vi "TIM Control GUI_Modified for Testing.vi"() -> ()   [LabVIEW 2018]
doc: "This example demonstrates how to use the PID Design function to obtain PID parameters based on measured process."
uses:
  <vilib>/DAQmx/write.llb/DAQmx Write (Digital 1D Bool 1Chan 1Samp).vi
  <vilib>/DAQmx/read.llb/DAQmx Read (Analog 1D DBL NChan 1Samp).vi
  <vilib>/Instr/_visa.llb/VISA Configure Serial Port (Instr).vi
  <vilib>/DAQmx/create/channels.llb/DAQmx Create Channel (DO-Digital Output).vi
  <vilib>/DAQmx/miscellaneous.llb/DAQmx Fill In Error Info.vi
  <vilib>/addons/control/pid/pid.llb/PID Advanced (DBL).vi
  <vilib>/addons/control/pid/autopid.llb/PID Autotuning Design (Ziegler-Nichols).vi
  <vilib>/addons/control/pid/autopid.llb/PID Autotuning Design (Cohen-Coon).vi
  <vilib>/addons/control/pid/autopid.llb/PID Autotuning Design (Chien-Hrones-Reswick).vi
  <vilib>/addons/control/pid/autopid.llb/PID Autotuning Design (Internal Model Control).vi
  <vilib>/addons/control/pid/NI_PID_autopid.lvlib
  <vilib>/addons/control/pid/NI_PID_pid.lvlib
  <vilib>/ptbypt/NI_PtbyPt.lvlib
panel:
  out "Tracker 4 - X,Y,Z":cluster{"x":sgl, "y":sgl, "z":sgl}(graph)
  out "Tracker 3 - X,Y,Z":cluster{"x":sgl, "y":sgl, "z":sgl}(graph)
  out "Tracker 2 - X,Y,Z":cluster{"x":sgl, "y":sgl, "z":sgl}(graph)
  out "Tracker 1 - X,Y,Z":cluster{"x":sgl, "y":sgl, "z":sgl}(graph)
  in  "Set Point 1,5":dbl
  out "Real time Data 1,5,3,4":dbl[][](graph)
  in  "Set Point 2":dbl
  out "Real time Data 2":dbl[][](graph)
  in  "Set Point 7":dbl
  out "Real time Data 7":dbl[][](graph)
  in  "Set Point  6,8,9,10":dbl
  out "Real time Data 6,8,9,10":dbl[][](graph)
  in  "Set Point 11,12":dbl
  out "Real time Data -11,12":dbl[][](graph)
  out "error out":errorcluster {"code" format="%.0x"}
  in  "XYZAER":T1(array[cluster]) {"r" format="%1_6f"; "e" format="%1_6f"; "a" format="%1_6f"; "z" format="%1_6f"; "y" format="%1_6f"; "x" format="%1_6f"}
  out "Start Time Text":string
  out "Stop Time Text":string
  out "Elapsed Time Text":string
  out "HostFrameCount":u32
  out "Loop Iter":i32
  out "PnoData":bool
  in  "stop":bool
  out "?":bool
  in  "Muscle Control":T2(tab)=enum."M-11,12"
  out "Tuned PID gains 12":T3={"proportional gain (Kc)"=1.9838195929127882, "integral time (Ti, min)"=0.01995856284686879, "derivative time (Td, min)"=0.0} {"derivative time (Td, min)" format="%#.6g"; "integral time (Ti, min)" format="%#.6g"; "proportional gain (Kc)" format="%#.6g"}
  in  "Accept gain 12":bool
  in  "Control 12":T4(tab)
  in  "Ziegler-Nichols speed 12":u16(ring) items=["Fast", "Normal", "Slow"]
  in  "Tuning specifications 12":u16(ring) items=["Regulator - 0 %", "Regulator -  20%", "Servo - 0%", "Servo - 20%"]
  in  "Multiplicative factor 12":dbl(slide)=1.0 scale=0.01..100.0
  in  "Type of controller 12":u16(ring)=2 items=["P", "PI", "PID"]
  in  "Stop 12":bool
  in  "PID Gains 12":T3={"proportional gain (Kc)"=0.1625, "integral time (Ti, min)"=1.25, "derivative time (Td, min)"=0.0} {"derivative time (Td, min)" format="%#.6g"; "integral time (Ti, min)" format="%#.6g"; "proportional gain (Kc)" format="%#.6g"}
  in  "Autotune 12":bool
  in  "Reinitialize 12":bool
  in  "Excitation 12":dbl=0.5 format="%.2f"
  in  "Automatic 12":bool=TRUE
  in  "MV: 12":dbl(slide)=20.39115328927357 scale=-100.0..100.0
  out "PWM Output 12":bool
  in  "Median sample length 21":i32=100
  in  "INLET 1,5 ON/OFF 3":bool=TRUE
  out "Tuned PID gains 8":T3={"proportional gain (Kc)"=1.9838195929127882, "integral time (Ti, min)"=0.01995856284686879, "derivative time (Td, min)"=0.0} {"derivative time (Td, min)" format="%#.6g"; "integral time (Ti, min)" format="%#.6g"; "proportional gain (Kc)" format="%#.6g"}
  in  "Accept gain 8":bool
  in  "Control 8":T4(tab)
  in  "Ziegler-Nichols speed 8":u16(ring) items=["Fast", "Normal", "Slow"]
  in  "Tuning specifications 8":u16(ring) items=["Regulator - 0 %", "Regulator -  20%", "Servo - 0%", "Servo - 20%"]
  in  "Multiplicative factor 8":dbl(slide)=1.0 scale=0.01..100.0
  in  "Type of controller 8":u16(ring)=2 items=["P", "PI", "PID"]
  in  "Stop 8":bool
  in  "PID Gains 8":T3={"proportional gain (Kc)"=0.1625, "integral time (Ti, min)"=1.25, "derivative time (Td, min)"=0.0} {"derivative time (Td, min)" format="%#.6g"; "integral time (Ti, min)" format="%#.6g"; "proportional gain (Kc)" format="%#.6g"}
  in  "Autotune 8":bool
  in  "Reinitialize 8":bool
  in  "Excitation 8":dbl=0.5 format="%.2f"
  in  "Automatic 8":bool=TRUE
  in  "MV: 8":dbl(slide)=20.39115328927357 scale=-100.0..100.0
  out "PWM Output 8":bool
  in  "Median sample length 17":i32=100
  in  "INLET 2 ON/OFF 2":bool=TRUE
  out "Tuned PID gains 7":T3={"proportional gain (Kc)"=1.9838195929127882, "integral time (Ti, min)"=0.01995856284686879, "derivative time (Td, min)"=0.0} {"derivative time (Td, min)" format="%#.6g"; "integral time (Ti, min)" format="%#.6g"; "proportional gain (Kc)" format="%#.6g"}
  in  "Accept gain 7":bool
  in  "Control 7":T4(tab)
  in  "Ziegler-Nichols speed 7":u16(ring) items=["Fast", "Normal", "Slow"]
  in  "Tuning specifications 7":u16(ring) items=["Regulator - 0 %", "Regulator -  20%", "Servo - 0%", "Servo - 20%"]
  in  "Multiplicative factor 7":dbl(slide)=1.0 scale=0.01..100.0
  in  "Type of controller 7":u16(ring)=2 items=["P", "PI", "PID"]
  in  "Stop 7":bool
  in  "PID Gains 7":T3={"proportional gain (Kc)"=0.1625, "integral time (Ti, min)"=1.25, "derivative time (Td, min)"=0.0} {"derivative time (Td, min)" format="%#.6g"; "integral time (Ti, min)" format="%#.6g"; "proportional gain (Kc)" format="%#.6g"}
  in  "Autotune 7":bool
  in  "Reinitialize 7":bool
  in  "Excitation 7":dbl=0.5 format="%.2f"
  in  "Automatic 7":bool=TRUE
  in  "MV: 7":dbl(slide)=20.39115328927357 scale=-100.0..100.0
  out "PWM Output 7":bool
  in  "Median sample length 16":i32=100
  in  "INLET 7 ON/OFF 2":bool=TRUE
  out "Tuned PID gains 6":T3={"proportional gain (Kc)"=1.9838195929127882, "integral time (Ti, min)"=0.01995856284686879, "derivative time (Td, min)"=0.0} {"derivative time (Td, min)" format="%#.6g"; "integral time (Ti, min)" format="%#.6g"; "proportional gain (Kc)" format="%#.6g"}
  in  "Accept gain 6":bool
  in  "Control 6":T4(tab)
  in  "Ziegler-Nichols speed 6":u16(ring) items=["Fast", "Normal", "Slow"]
  in  "Tuning specifications 6":u16(ring) items=["Regulator - 0 %", "Regulator -  20%", "Servo - 0%", "Servo - 20%"]
  in  "Multiplicative factor 6":dbl(slide)=1.0 scale=0.01..100.0
  in  "Type of controller 6":u16(ring)=2 items=["P", "PI", "PID"]
  in  "Stop 6":bool
  in  "PID Gains 6":T3={"proportional gain (Kc)"=0.1625, "integral time (Ti, min)"=1.25, "derivative time (Td, min)"=0.0} {"derivative time (Td, min)" format="%#.6g"; "integral time (Ti, min)" format="%#.6g"; "proportional gain (Kc)" format="%#.6g"}
  in  "Autotune 6":bool
  in  "Reinitialize 6":bool
  in  "Excitation 6":dbl=0.5 format="%.2f"
  in  "Automatic 6":bool=TRUE
  in  "MV: 6":dbl(slide)=20.39115328927357 scale=-100.0..100.0
  out "PWM Output 6":bool
  in  "Median sample length 15":i32=100
  in  "INLET 6 ON/OFF 2":bool=TRUE
  in  "INLET":bool=TRUE
  out "PWM Output":bool
  in  "MV:":dbl(slide)=20.39115328927357 scale=-100.0..100.0
  in  "Median sample length":i32=100
  in  "Excitation":dbl=0.5 format="%.2f"
  in  "Type of controller":u16(ring)=2 items=["P", "PI", "PID"]
  in  "Control":T4(tab)
  in  "Ziegler-Nichols speed":u16(ring) items=["Fast", "Normal", "Slow"]
  in  "Tuning specifications":u16(ring) items=["Regulator - 0 %", "Regulator -  20%", "Servo - 0%", "Servo - 20%"]
  in  "Multiplicative factor":dbl(slide)=1.0 scale=0.01..100.0
  in  "Automatic":bool=TRUE
  in  "Reinitialize":bool
  in  "Accept gain":bool
  out "Tuned PID gains":T3={"proportional gain (Kc)"=1.9838195929127882, "integral time (Ti, min)"=0.01995856284686879, "derivative time (Td, min)"=0.0} {"derivative time (Td, min)" format="%#.6g"; "integral time (Ti, min)" format="%#.6g"; "proportional gain (Kc)" format="%#.6g"}
  in  "Autotune":bool
  in  "PID Gains":T3={"proportional gain (Kc)"=0.1625, "integral time (Ti, min)"=1.25, "derivative time (Td, min)"=0.0} {"derivative time (Td, min)" format="%#.6g"; "integral time (Ti, min)" format="%#.6g"; "proportional gain (Kc)" format="%#.6g"}
  in  "Stop":bool
  in  "M-11,12":i32=5
  in  "M-6,8,9,10":i32=5
  in  "M-7":i32=5
  in  "M-2":i32=5
  in  "M-1,5":i32=5
  out "Stimulus operating point 12":dbl=20.314221540357543
  out "Response operating point 12":dbl=51.08345461694337
  out "Identified Plant Parameters 12":T5={"Plant Gain (K)"=1.7609511324977591, "Time Constant (T)"=1.9621978490901302, "Dead Time (L)"=0.22467425343567116}
  out "Control Output 12":dbl[](graph)
  out "Measurement 12":dbl[](graph)
  out "Identified Plant Parameters":T5={"Plant Gain (K)"=1.7609511324977591, "Time Constant (T)"=1.9621978490901302, "Dead Time (L)"=0.22467425343567116}
  out "Control Output":dbl[](graph)
  out "Measurement":dbl[](graph)
  out "Stimulus operating point":dbl=20.314221540357543
  out "Response operating point":dbl=51.08345461694337
  out "Stimulus operating point 6":dbl=20.314221540357543
  out "Response operating point 6":dbl=51.08345461694337
  out "Identified Plant Parameters 6":T5={"Plant Gain (K)"=1.7609511324977591, "Time Constant (T)"=1.9621978490901302, "Dead Time (L)"=0.22467425343567116}
  out "Control Output 6":dbl[](graph)
  out "Measurement 6":dbl[](graph)
  out "Stimulus operating point 7":dbl=20.314221540357543
  out "Response operating point 7":dbl=51.08345461694337
  out "Identified Plant Parameters 7":T5={"Plant Gain (K)"=1.7609511324977591, "Time Constant (T)"=1.9621978490901302, "Dead Time (L)"=0.22467425343567116}
  out "Control Output 7":dbl[](graph)
  out "Measurement 7":dbl[](graph)
  out "Stimulus operating point 8":dbl=20.314221540357543
  out "Response operating point 8":dbl=51.08345461694337
  out "Identified Plant Parameters 8":T5={"Plant Gain (K)"=1.7609511324977591, "Time Constant (T)"=1.9621978490901302, "Dead Time (L)"=0.22467425343567116}
  out "Control Output 8":dbl[](graph)
  out "Measurement 8":dbl[](graph)
  out "Connected":bool
  out "Running":bool
  out "Position Sensor Data":cluster{dbl, "x":sgl}[](graph)
  out "Sensor Raw Value 2":i32
  in  "COM Port-Sensor 2":refnum<visa-resource-name>="COM5"
  in  "upper/lower infle":enum32{"Page 1", "Page 2"}(tab)
  out "Force in Kilograms":dbl(graph)
  out "Force in Newtons":dbl(graph)
  in  "lower/upper infle":enum32{"Page 1", "Page 2"}(tab)
  out "Force in Newtons 2":dbl(graph)
  out "Force in Kilograms 2":dbl(graph)
  in  "COM Port-Sensor 1":refnum<visa-resource-name>="COM4"
  out "Sensor Raw Value":i32
  in  "Tab Control":T6(tab)
  in  "Instructions":string="Overview: This example demonstrates how to use the PID Autotuning Design to obtain PID parameters based on setpoint and process variable collected in another loop.\nInstructions:\n1. Run the VI and wait until the process variable (PV) reaches near setpoint (SP).\n2.  In the PID Autotuning Design section, select the type of algorithm, type of controller and excitation amplitude for the 'open loop step response'. Then, click Autotune to start the process. Select the Identified Plant Parameter tab and see the results from the identification.\n3.  When the tuned PID gains do not change anymore, the identification is done and you have the option to accept by clicking Accept gain, which will transfer the new gain to PID Gains.\n4. Click the Autotune button again to go back to the automatic control state. You can try different options and repeat this process.\n5. Click Stop to stop the VI.\n"
  # "Pressure Alarm"
  # "Force Sensor Data"
  # "Position Sensor Data"
  # "PID Controller"
  # "PID Autotuning Design"
  # "No additional parameters"
  # "PID Controller"
  # "PID Autotuning Design"
  # "PID Controller"
  # "PID Autotuning Design"
  # "No additional parameters"
  # "PID Controller"
  # "PID Autotuning Design"
  # "No additional parameters"
  # "PID Controller"
  # "PID Autotuning Design"
  # "No additional parameters"
  # "Muscle Control"
  # "PID Controller"
  # "PID Autotuning Design"
  # "No additional parameters"
  # "Pressure Cut Off to trigger the alarm"
  # "M-11,12"
  # "M-3,4"
  # "M-1,5"
  # "M-6,8,9,10"
  # "M-7"
  # "M-2"
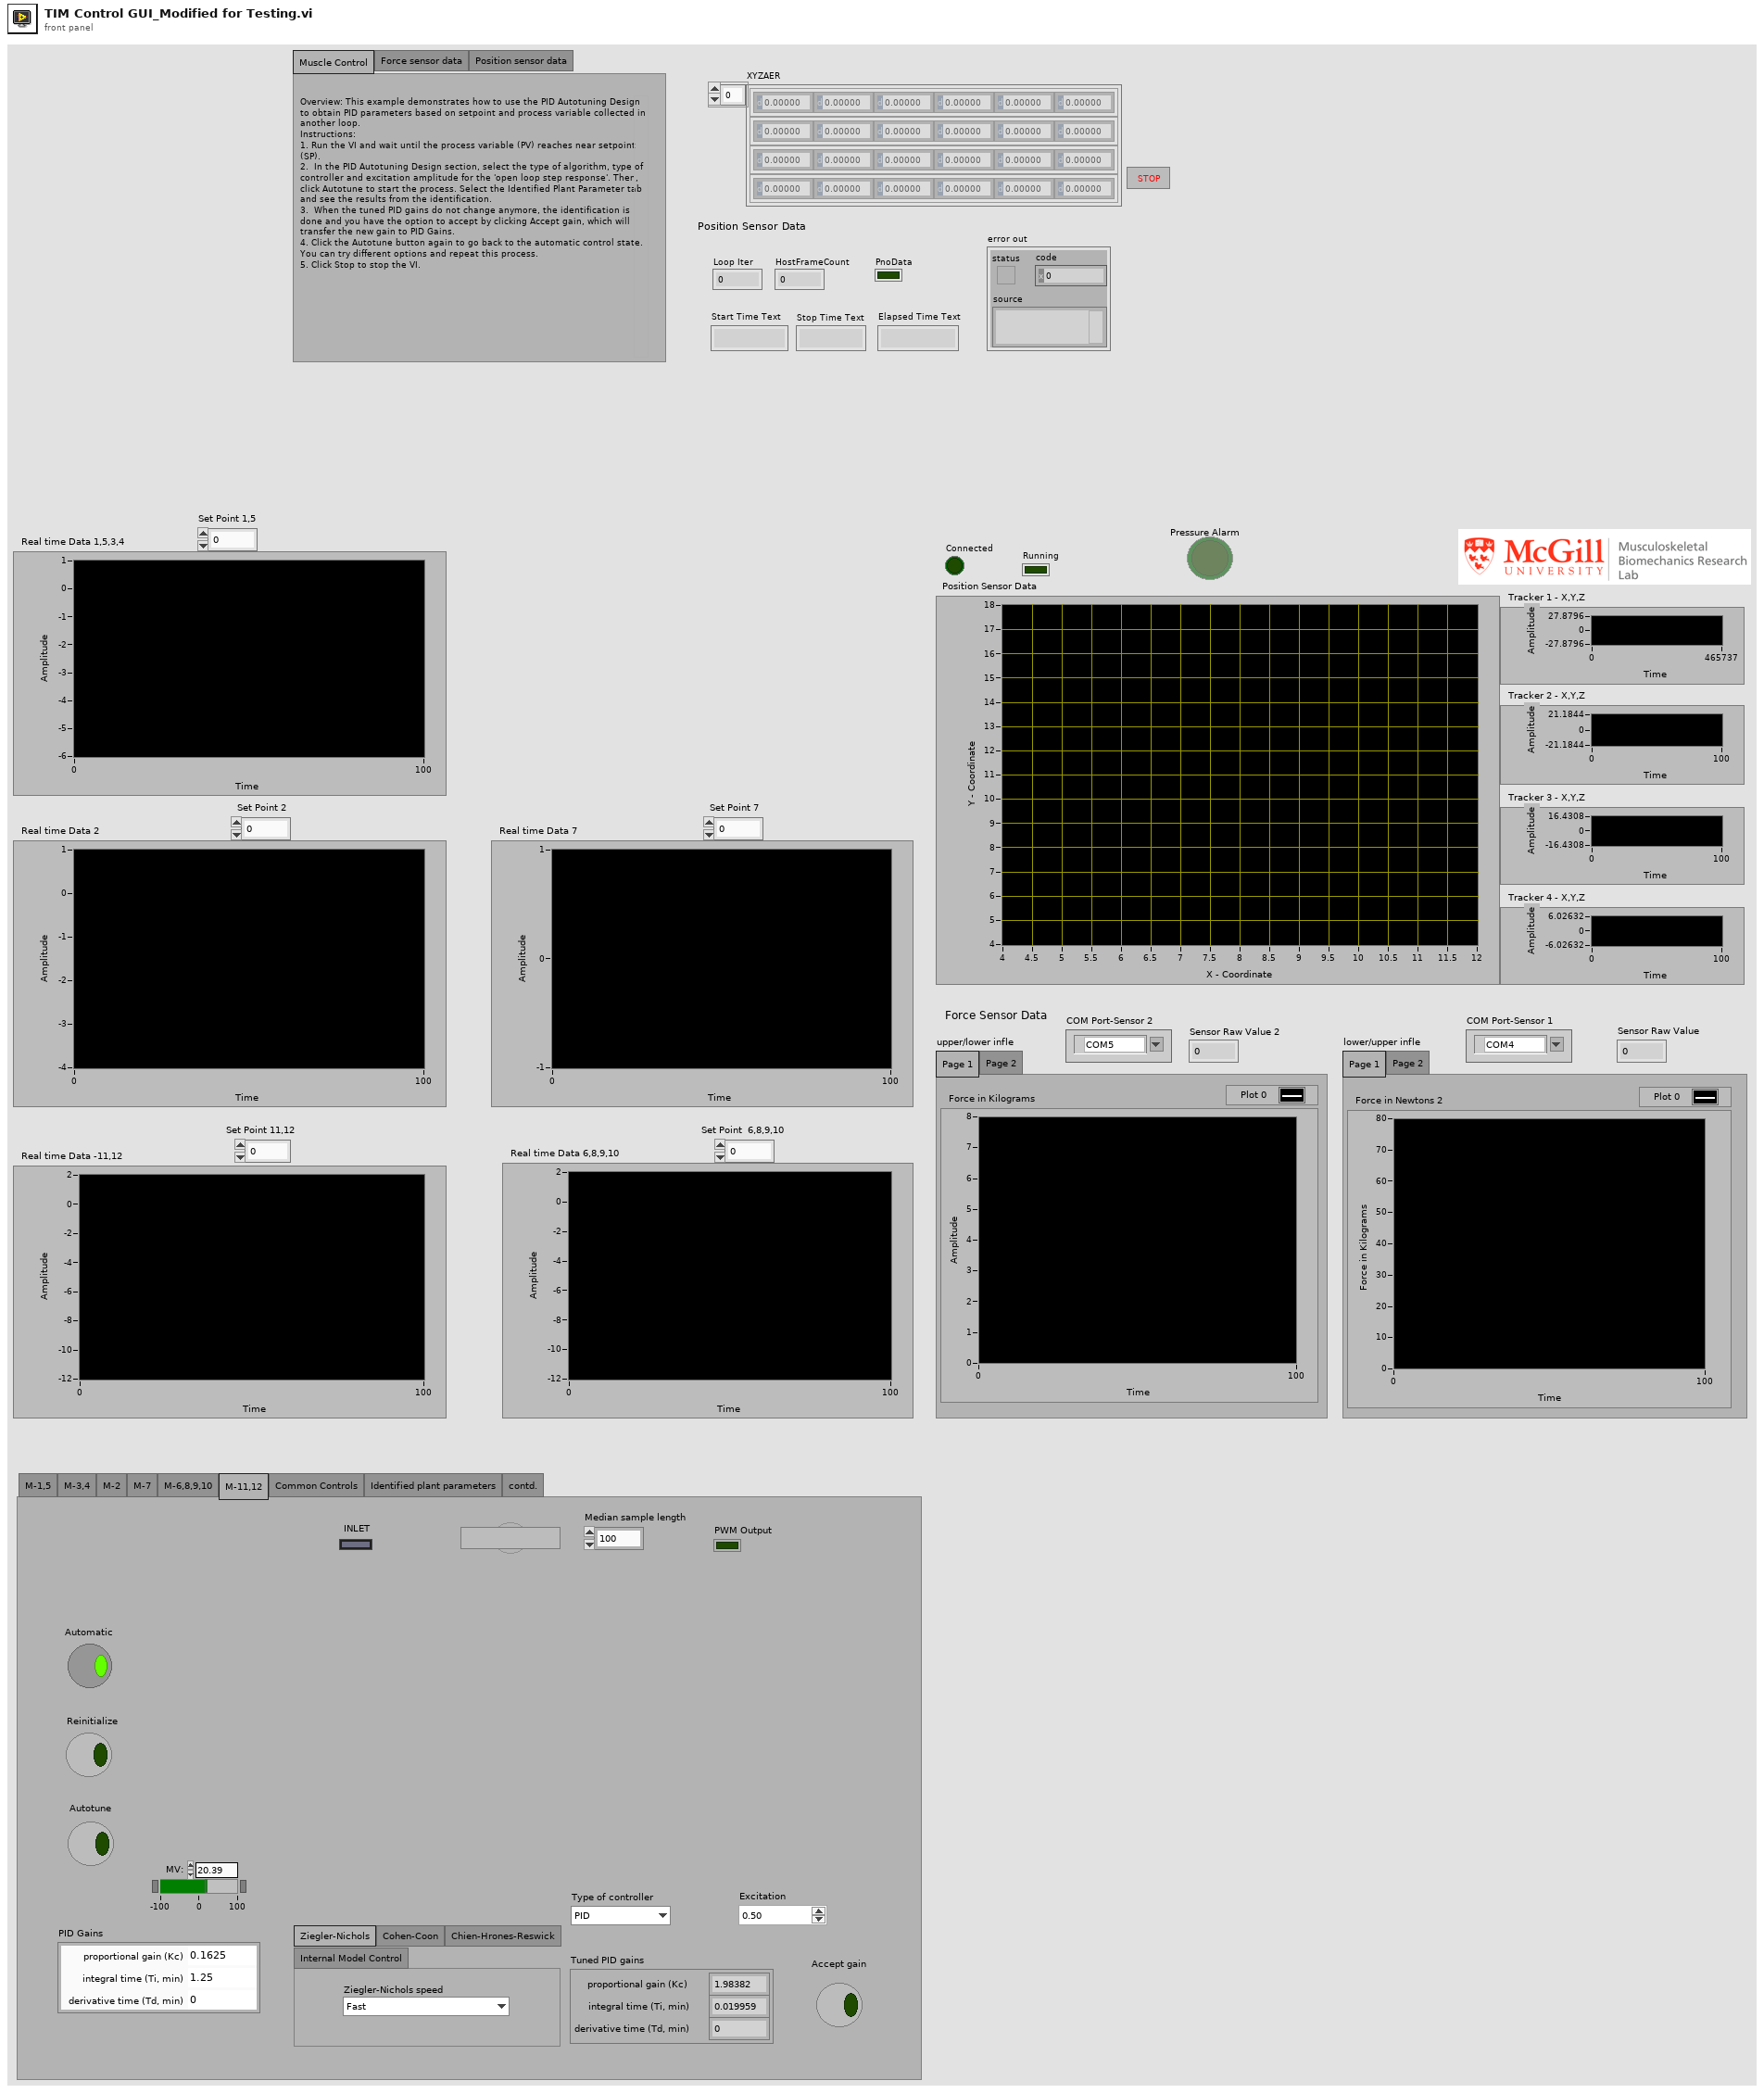
[diagram p1: front panel]
types:
  T1 = cluster{"x":sgl, "y":sgl, "z":sgl, "a":sgl, "e":sgl, "r":sgl}[]
  T2 = enum32{"M-1,5", "M-3,4", "M-2", "M-7", "M-6,8,9,10", "M-11,12", "Common Controls", "Identified plant parameters", "contd."}
  T3 = cluster{"proportional gain (Kc)":dbl, "integral time (Ti, min)":dbl, "derivative time (Td, min)":dbl}
  T4 = enum32{"Ziegler-Nichols", "Cohen-Coon", "Chien-Hrones-Reswick", "Internal Model Control"}
  T5 = cluster{"Plant Gain (K)":dbl, "Time Constant (T)":dbl, "Dead Time (L)":dbl}
  T6 = enum32{"Muscle Control", "Force sensor data", "Position sensor data"}
  T7 = cluster{"static gain":dbl, "lag (s)":dbl, "deadtime (s)":dbl, "load":dbl, "deadband":dbl, "sensor noise":dbl, "initial PV":dbl, "plant noise":dbl}
  T8 = cluster{"x":sgl, "y":sgl, "z":sgl, "a":sgl, "e":sgl, "r":sgl}
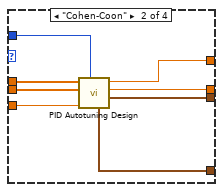
[diagram p2: hidden frame]
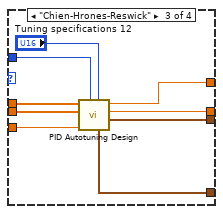
[diagram p3: hidden frame]
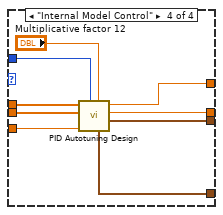
[diagram p4: hidden frame]
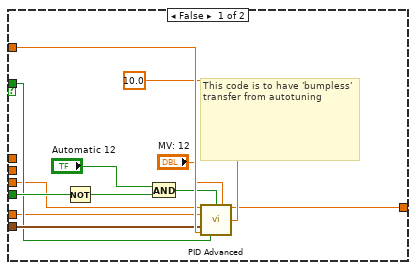
[diagram p6: hidden frame]
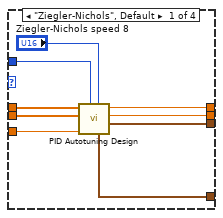
[diagram p7: hidden frame]
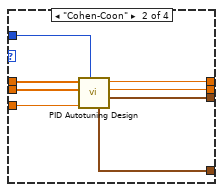
[diagram p8: hidden frame]
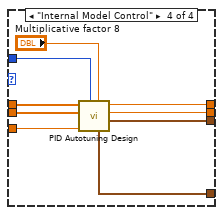
[diagram p9: hidden frame]
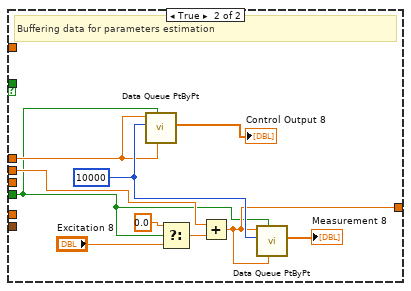
[diagram p11: hidden frame]
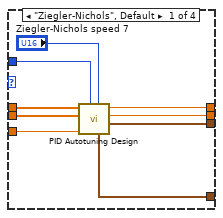
[diagram p12: hidden frame]
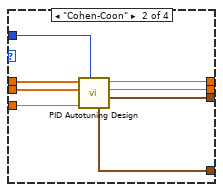
[diagram p13: hidden frame]
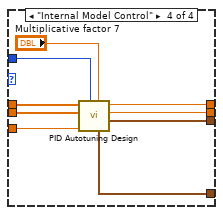
[diagram p14: hidden frame]
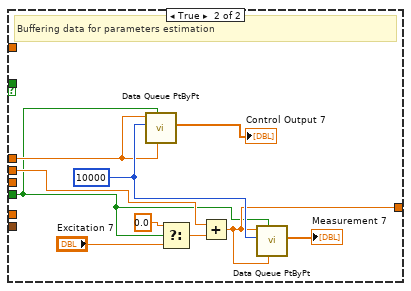
[diagram p16: hidden frame]
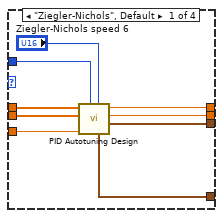
[diagram p17: hidden frame]
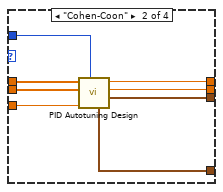
[diagram p18: hidden frame]
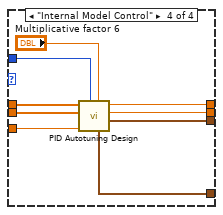
[diagram p19: hidden frame]
diagram:
  w16 = 0.0 ("output")
  w19 = FALSE ("Stop")
  w22 = 0.0 ("output")
  w25 = FALSE ("Stop")
  w28 = 0.0 ("output")
  w31 = FALSE ("Stop")
  w34 = 0.0 ("output")
  w37 = FALSE ("Stop")
  w42 = 2400  # BufferFrameCount
  w76 = 0.0 ("output")
  w79 = FALSE ("Stop")
  # "Muscle-1,5 PID CONTROL LOOP (Auto Tuning)"
  # "Muscle-2 PID CONTROL LOOP (Auto Tuning)"
  # "Muscle-7 PID CONTROL LOOP (Auto Tuning)"
  # "Muscle-6,8,9,10 PID CONTROL LOOP (Auto Tuning)"
  # "Muscle-11,12 PID CONTROL LOOP (Auto Tuning)"
  # "FORCE SENSOR CONTROL LOOP"
  # "POSITION SENSOR CONTROL LOOP"
  # "Pressure Alarm"
  # "8. Close Tracker connection."
  # "3. Query Max num sensors supported by the tracker."
  # "4. Allocate raw buffer to hold 2400 frames of data."
  # "5. Start Continuous mode."
  # "7. Stop Continuous mode."
  # "6. Start the loop. Loop exits when Stop Button is hit."
  n1 = Obtain Queue(element data type=0.0) -> (queue out=w11:refnum<queue>)  [unwired: 4 in, 2 out]
  n2 = while {
    shift-left: 0.0 ("Plant Output") -> [w195]
    shift-right: [w190] -> _
    tunnel: w37 -> [_]
    shift-right: [w176] -> _
    shift-left: 0.01 -> [w174]
    shift-right: [w149] -> _
    shift-left: TRUE -> [w173]
    shift-right: [w151] -> _
    shift-left: w34 -> [w172]
    shift-right: [w175] -> _
    shift-left: w34 -> [w171]
    tunnel: [w146] -> w33
    tunnel: [w133] -> w3
    tunnel: w11 -> [w131]
    stop <- "Stop 6" stop-if-true
    w84 = 1 items=["one channel for each line", "one channel for all lines"] ("line grouping")
    w92 = 1 items=["one channel for each line", "one channel for all lines"] ("line grouping")
    w100 = 1 items=["one channel for each line", "one channel for all lines"] ("line grouping")
    w108 = 1 items=["one channel for each line", "one channel for all lines"] ("line grouping")
    w116 = 1 items=["one channel for each line", "one channel for all lines"] ("line grouping")
    w124 = 1 items=["one channel for each line", "one channel for all lines"] ("line grouping")
    w137 = 1 items=["one channel for each line", "one channel for all lines"] ("line grouping")
    w146 = 0.05 ("Sampling Time dt (s)")
    w154 = 1 items=["one channel for each line", "one channel for all lines"] ("line grouping")
    w162 = 0.5 ("x")
    w189 = T7 {"static gain"=2.5, "lag (s)"=2.5, "deadtime (s)"=0.01, "load"=0.0, "deadband"=0.0, "sensor noise"=0.0, "initial PV"=30.0, "plant noise"=0.0}  # Process parameters
    w191 = FALSE  # Integrator ?
    # "Inlet 11"
    # "Exhaust 10"
    # "Inlet 11"
    # "Exhaust 9"
    # "Inlet 11"
    # "Exhaust 8"
    # "C."
    # "Inlet 11"
    # "Exhaust 6"
    # "B."
    # "A."
    # "A.Output to PWM Logic \nB. Simulated Plant\nC. Draw Chart"
    # "Main PID Loop Control"
    n3 = Dequeue Element(queue=w131) -> (element=w132:dbl)  [unwired: 2 in, 3 out]
    n4 = Multiply(x=w146, y=1000.0) -> (x*y=w188:dbl)
    n5 = Not(x="Autotune 6") -> (.not. x?=w192:bool)
    n6 = feedback #1() -> (w197:bool)  [unwired: 1 in]
    n7 = feedback-in #1("Autotune 6") -> ()
    n8 = Wait Until Next ms Multiple(millisecond multiple=w188) -> ()  [unwired: 1 out]
    n9 = Exclusive Or(1:w197, 2:"Autotune 6") -> (0:w196:bool)
    n10 = feedback #2() -> (w194:dbl)  [unwired: 1 in]
    n11 = Multiply(x=w132, y=-1000.0) -> (x*y=w178:dbl)
    n12 = call <vilib>:"Median PtByPt.vi"("sample length"="Median sample length 15", "x"=w178) -> ("median"=w177:dbl)  [unwired: 2 in, 1 out]
    n13 = Square(x=w177) -> (x^2=w185:dbl)
    n14 = Multiply(x=w177, y=16.572) -> (x*y=w181:dbl)
    n15 = Multiply(x=w185, y=-0.06) -> (x*y=w182:dbl)
    n16 = Add(x=w181, y=w182) -> (x+y=w180:dbl)
    n17 = Add(x=-1011.3, y=w180) -> (x+y=w144:dbl)
    n18 = case shown="False" "Autotune 6" {
      tunnel: w146 -> [w212 _]
      tunnel: [w201 w217] -> w151
      tunnel: w195 -> [_ w216]
      tunnel: "PID Gains 6" -> [w211 _]
      tunnel: "Reinitialize 6" -> [w208 _]
      tunnel: w196 -> [w210 w215]
      tunnel: w194 -> [_ w219]
      tunnel: w144 -> [w204 _]
      tunnel: "Set Point  6,8,9,10" -> [w203 _]
      frame False {
        # "This code is to have 'bumpless' transfer from autotuning"
        n19 = Not(x=w210) -> (.not. x?=w207:bool)
        n20 = And(x="Automatic 6", y=w207) -> (x .and. y?=w209:bool)
        n21 = call-poly <vilib>:"PID Advanced.vi"("setpoint"=w203, "auto? (T)"=w209, "manual control"="MV: 6", "process variable"=w204, "alpha"=10.0, "PID gains"=w211, "dt (s)"=w212, "reinitialize? (F)"=w208) -> ("output"=w201:dbl)  [unwired: 6 in, 1 out]
      }
      frame True {
        w222 = 10000 ("sample length")
        # "Buffering data for parameters estimation"
        n22 = call <vilib>:"Data Queue PtByPt.vi"("initial queue element"=w216, "initialize"=w215, "sample length"=w222, "input data point"=w216) -> ("Current Queue"=→"Control Output 6":dbl[])  [unwired: 3 in, 4 out]
        n23 = Select(t=0.0, s=w215, f="Excitation 6") -> (s? t:f=w220:dbl)
        n24 = Add(x=w219, y=w220) -> (x+y=w217:dbl)
        n25 = call <vilib>:"Data Queue PtByPt.vi"("initial queue element"=w217, "initialize"=w215, "sample length"=w222, "input data point"=w217) -> ("Current Queue"=→"Measurement 6":dbl[])  [unwired: 3 in, 4 out]
      }
    }
    n26 = feedback-in #2(w151, w192) -> ()
    n27 = Greater?(x=w144, y="M-6,8,9,10") -> (0:w133:bool)
    n28 = Add(x=w174, y=w162) -> (x+y=w163:dbl)
    n29 = Subtract(x=w174, y=w162) -> (x-y=w161:dbl)
    n30 = Equal?(x=w172, y=w151) -> (x = y?=w169:bool)
    n31 = Greater?(x=w151, y=w172) -> (0:w168:bool)
    n32 = Select(t=w173, s=w169, f=w168) -> (s? t:f=w149:bool)
    "PWM Output 6" <- w149
    n33 = call "Plant System.vi"("Integrator ?"=w191, "Plant Input"=w151, "dt (s)"=w146, "process parameters"=w189) -> ("Plant Output"=w190:dbl)  [unwired: 11 in]
    n34 = Increment(x="Set Point  6,8,9,10") -> (x+1=w167:dbl)
    n35 = Decrement(x="Set Point  6,8,9,10") -> (x-1=w166:dbl)
    n36 = Select(t=w163, s=w149, f=w161) -> (s? t:f=w176:dbl)
    n37 = call-poly <vilib>:"DAQmx Create Virtual Channel.vi"("lines"=tag "cDAQ1Mod1/port0/line3", "line grouping"=w108) -> ("task out"=w110:refnum<k21>, "error out"=w109:errorcluster)  [unwired: 12 in]
    n38 = call-poly <vilib>:"DAQmx Create Virtual Channel.vi"("lines"=tag "cDAQ1Mod2/port0/line3", "line grouping"=w100) -> ("task out"=w102:refnum<k21>, "error out"=w101:errorcluster)  [unwired: 12 in]
    n39 = Select(t=w167, s=w149, f=w166) -> (s? t:f=w165:dbl)
    n40 = Not(x=w149) -> (.not. x?=w148:bool)
    n41 = call-poly <vilib>:"DAQmx Create Virtual Channel.vi"("lines"=tag "cDAQ1Mod1/port0/line4", "line grouping"=w154) -> ("task out"=w156:refnum<k21>, "error out"=w155:errorcluster)  [unwired: 12 in]
    n42 = call-poly <vilib>:"DAQmx Create Virtual Channel.vi"("lines"=tag "cDAQ1Mod2/port0/line4", "line grouping"=w137) -> ("task out"=w139:refnum<k21>, "error out"=w138:errorcluster)  [unwired: 12 in]
    n43 = Build Array(w144, "Set Point  6,8,9,10", w165) -> (w164:dbl[])
    n44 = Initialize Array("INLET 6 ON/OFF 2", 1 ("dimension size")) -> (w81:bool[])
    n45 = Initialize Array(w148, 1 ("dimension size")) -> (w82:bool[])
    n46 = local write "MV: 6"(w151) -> ()
    n47 = Add(x=w171, y=w174) -> (x+y=w175:dbl)
    n48 = Build Array(w164) -> (→"Real time Data 6,8,9,10":dbl[][])
    n49 = call-poly <vilib>:"DAQmx Write.vi"("task/channels in"=w110, "auto start"=TRUE, "data"=w82, "error in"=w109) -> ("task out"=w112:refnum<k21>, "error out"=w113:errorcluster)  [unwired: 9 in, 1 out]
    n50 = call-poly <vilib>:"DAQmx Write.vi"("task/channels in"=w102, "auto start"=TRUE, "data"=w81, "error in"=w101) -> ("task out"=w104:refnum<k21>, "error out"=w105:errorcluster)  [unwired: 9 in, 1 out]
    n51 = call-poly <vilib>:"DAQmx Write.vi"("task/channels in"=w156, "auto start"=TRUE, "data"=w82, "error in"=w155) -> ("task out"=w158:refnum<k21>, "error out"=w159:errorcluster)  [unwired: 9 in, 1 out]
    n52 = call-poly <vilib>:"DAQmx Write.vi"("task/channels in"=w139, "auto start"=TRUE, "data"=w81, "error in"=w138) -> ("task out"=w141:refnum<k21>, "error out"=w142:errorcluster)  [unwired: 9 in, 1 out]
    n53 = call <vilib>:"DAQmx Clear Task.vi"("task in"=w112, "error in"=w113) -> ("error out"=w107:errorcluster)  [unwired: 13 in]
    n54 = call <vilib>:"DAQmx Clear Task.vi"("task in"=w104, "error in"=w105) -> ("error out"=w99:errorcluster)  [unwired: 13 in]
    n55 = call <vilib>:"DAQmx Clear Task.vi"("task in"=w158, "error in"=w159) -> ("error out"=w153:errorcluster)  [unwired: 13 in]
    n56 = call <vilib>:"DAQmx Clear Task.vi"("task in"=w141, "error in"=w142) -> ("error out"=w136:errorcluster)  [unwired: 13 in]
    n57 = call <vilib>:"Simple Error Handler.vi"("error in (no error)"=w107) -> ()  [unwired: 4 in, 5 out]
    n58 = call <vilib>:"Simple Error Handler.vi"("error in (no error)"=w99) -> ()  [unwired: 4 in, 5 out]
    n59 = call <vilib>:"Simple Error Handler.vi"("error in (no error)"=w153) -> ()  [unwired: 4 in, 5 out]
    n60 = call <vilib>:"Simple Error Handler.vi"("error in (no error)"=w136) -> ()  [unwired: 4 in, 5 out]
    n61 = call-poly <vilib>:"DAQmx Create Virtual Channel.vi"("lines"=tag "cDAQ1Mod8/port0/line6", "line grouping"=w92) -> ("task out"=w94:refnum<k21>, "error out"=w93:errorcluster)  [unwired: 12 in]
    n62 = call-poly <vilib>:"DAQmx Create Virtual Channel.vi"("lines"=tag "cDAQ1Mod7/port0/line5", "line grouping"=w84) -> ("task out"=w86:refnum<k21>, "error out"=w85:errorcluster)  [unwired: 12 in]
    n63 = call-poly <vilib>:"DAQmx Create Virtual Channel.vi"("lines"=tag "cDAQ1Mod8/port0/line3", "line grouping"=w124) -> ("task out"=w126:refnum<k21>, "error out"=w125:errorcluster)  [unwired: 12 in]
    n64 = call-poly <vilib>:"DAQmx Create Virtual Channel.vi"("lines"=tag "cDAQ1Mod7/port0/line2", "line grouping"=w116) -> ("task out"=w118:refnum<k21>, "error out"=w117:errorcluster)  [unwired: 12 in]
    n65 = call-poly <vilib>:"DAQmx Write.vi"("task/channels in"=w94, "auto start"=TRUE, "data"=w82, "error in"=w93) -> ("task out"=w96:refnum<k21>, "error out"=w97:errorcluster)  [unwired: 9 in, 1 out]
    n66 = call-poly <vilib>:"DAQmx Write.vi"("task/channels in"=w86, "auto start"=TRUE, "data"=w81, "error in"=w85) -> ("task out"=w88:refnum<k21>, "error out"=w89:errorcluster)  [unwired: 9 in, 1 out]
    n67 = call-poly <vilib>:"DAQmx Write.vi"("task/channels in"=w126, "auto start"=TRUE, "data"=w82, "error in"=w125) -> ("task out"=w128:refnum<k21>, "error out"=w129:errorcluster)  [unwired: 9 in, 1 out]
    n68 = call-poly <vilib>:"DAQmx Write.vi"("task/channels in"=w118, "auto start"=TRUE, "data"=w81, "error in"=w117) -> ("task out"=w120:refnum<k21>, "error out"=w121:errorcluster)  [unwired: 9 in, 1 out]
    n69 = call <vilib>:"DAQmx Clear Task.vi"("task in"=w96, "error in"=w97) -> ("error out"=w91:errorcluster)  [unwired: 13 in]
    n70 = call <vilib>:"DAQmx Clear Task.vi"("task in"=w88, "error in"=w89) -> ("error out"=w83:errorcluster)  [unwired: 13 in]
    n71 = call <vilib>:"DAQmx Clear Task.vi"("task in"=w128, "error in"=w129) -> ("error out"=w123:errorcluster)  [unwired: 13 in]
    n72 = call <vilib>:"DAQmx Clear Task.vi"("task in"=w120, "error in"=w121) -> ("error out"=w115:errorcluster)  [unwired: 13 in]
    n73 = call <vilib>:"Simple Error Handler.vi"("error in (no error)"=w91) -> ()  [unwired: 4 in, 5 out]
    n74 = call <vilib>:"Simple Error Handler.vi"("error in (no error)"=w83) -> ()  [unwired: 4 in, 5 out]
    n75 = call <vilib>:"Simple Error Handler.vi"("error in (no error)"=w123) -> ()  [unwired: 4 in, 5 out]
    n76 = call <vilib>:"Simple Error Handler.vi"("error in (no error)"=w115) -> ()  [unwired: 4 in, 5 out]
  }
  n77 = local write "Stop 6"(w37) -> ()
  n78 = while {
    tunnel: w37 -> [_]
    tunnel: w33 -> [w226]
    stop <- w236 stop-if-true
    # "If dT and deadtime have similar values, the identification could evaluate deadtime as zero and this generates proportional gain equal to Inf. This code avoid gain changes in this situations."
    # "Autotuning Loop"
    n79 = local read "Control Output 6"() -> (w238:dbl[])
    n80 = local read "Measurement 6"() -> (w237:dbl[])
    n81 = case shown="\"Chien-Hrones-Reswick\"" "Control 6" {
      tunnel: w238 -> [w247 w255 w264 w273]
      tunnel: w237 -> [w246 w254 w263 w272]
      tunnel: [w245 w253 w262 w271] -> w225
      tunnel: [w244 w252 w261 w270] -> w224
      tunnel: w226 -> [w243 w251 w260 w269]
      tunnel: [w242 w250 w259 w268] -> w223
      tunnel: [w241 w249 w258 w267] -> w228
      tunnel: "Type of controller 6" -> [w240 w248 w257 w266]
      frame "Ziegler-Nichols", Default {
        n82 = call-poly <vilib>:"PID Autotuning Design.vi"("Ziegler-Nichols Speed"="Ziegler-Nichols speed 6", "Type of Controller"=w240, "dt (s)"=w243, "Response signal"=w246, "Stimulus signal"=w247) -> ("PID gains"=w241:T3, "response operating point"=w244:dbl, "stimulus operating point"=w245:dbl, "Plant Parameters"=w242:T5)  [unwired: 3 in]
      }
      frame "Cohen-Coon" {
        n83 = call-poly <vilib>:"PID Autotuning Design.vi"("Type of Controller"=w248, "dt (s)"=w251, "Response signal"=w254, "Stimulus signal"=w255) -> ("PID gains"=w249:T3, "response offset"=w252:dbl, "stimulus offset"=w253:dbl, "Plant Parameters"=w250:T5)  [unwired: 4 in]
      }
      frame "Chien-Hrones-Reswick" {
        n84 = call-poly <vilib>:"PID Autotuning Design.vi"("Tuning specifications"="Tuning specifications 6", "Type of Controller"=w257, "dt (s)"=w260, "Response signal"=w263, "Stimulus signal"=w264) -> ("PID gains"=w258:T3, "response offset"=w261:dbl, "stimulus offset"=w262:dbl, "Plant Parameters"=w259:T5)  [unwired: 3 in]
      }
      frame "Internal Model Control" {
        n85 = call-poly <vilib>:"PID Autotuning Design.vi"("Desired Time Constant (tau_c)"="Multiplicative factor 6", "Type of Controller"=w266, "dt (s)"=w269, "Response signal"=w272, "Stimulus signal"=w273) -> ("PID gains"=w267:T3, "response offset"=w270:dbl, "stimulus offset"=w271:dbl, "Plant Parameters"=w268:T5)  [unwired: 3 in]
      }
    }
    "Stimulus operating point 6" <- w225
    "Response operating point 6" <- w224
    "Identified Plant Parameters 6" <- w223
    n86 = Unbundle(w228) -> ("proportional gain (Kc)"=w231:dbl)  [unwired: 2 out]
    n87 = Equal?(x=w231, y=inf) -> (x = y?=w230:bool)
    n88 = feedback #3() -> (w229:T3)  [unwired: 1 in]
    n89 = Select(t=w229, s=w230, f=w228) -> (s? t:f=w227:T3)
    "Tuned PID gains 6" <- w227
    n90 = feedback-in #3(w227) -> ()
    n91 = case shown="True" "Accept gain 6" {
      tunnel: w227 -> [_ w274]
      frame False {
      }
      frame True {
        n92 = local write "PID Gains 6"(w274) -> ()
      }
    }
    n93 = local read "Stop 6"() -> (w236:bool)
  }
  n94 = local write "Stop"(w79) -> ()
  n95 = call-poly "VISA Configure Serial Port"("VISA resource name"="COM Port-Sensor 1") -> ("VISA resource name out"=w70:refnum<visa-resource-name>, "error out"=w69:errorcluster)  [unwired: 9 in, 4 out]
  n96 = call-poly "VISA Configure Serial Port"("VISA resource name"="COM Port-Sensor 2") -> ("VISA resource name out"=w65:refnum<visa-resource-name>, "error out"=w64:errorcluster)  [unwired: 9 in, 4 out]
  n97 = while {
    shift-right: [w282] -> w71
    shift-left: w70 -> [w278]
    tunnel: w69 -> [w277]
    tunnel: [w279] -> w72
    stop <- w280 stop-if-true
    # "Serial Read Loop"
    n98 = case shown="True" TRUE {
      tunnel: [w294 w298] -> w282
      tunnel: w278 -> [w296 w298]
      tunnel: [w293 w297] -> w279
      tunnel: w277 -> [w295 w297]
      frame True {
        n99 = VISA Read(VISA resource name=w296, byte count=u32 1000, error in (no error)=w295) -> (VISA resource name out=w294:refnum<visa-resource-name>, read buffer=w291:string, error out=w293:errorcluster)  [unwired: 1 out]
        n100 = Decimal String To Number(string=w291) -> (number=w289:i32)  [unwired: 2 in, 1 out]
        "Sensor Raw Value" <- w289
        n101 = call <vilib>:"Median PtByPt.vi"("sample length"=20, "x"=w289) -> ("median"=w287:dbl)  [unwired: 2 in, 1 out]
        n102 = To Double Precision Float(number=w287) -> (double precision float=w283:dbl)
        n103 = Multiply(x=w283, y=0.0292) -> (x*y=w286:dbl)
        "Force in Kilograms 2" <- w286
        n104 = Multiply(x=w286, y=9.81) -> (x*y=→"Force in Newtons 2":dbl)
      }
      frame False {
      }
    }
    n105 = Wait (ms)(milliseconds to wait=u32 5) -> ()  [unwired: 1 out]
    n106 = Or(x=w279, y=FALSE) -> (x .or. y?=w280:bool)
  }
  n107 = while {
    shift-right: [w306] -> w39
    shift-left: w65 -> [w302]
    tunnel: w64 -> [w301]
    tunnel: [w303] -> w66
    stop <- w304 stop-if-true
    # "Serial Read Loop"
    n108 = case shown="True" TRUE {
      tunnel: [w318 w322] -> w306
      tunnel: w302 -> [w320 w322]
      tunnel: [w317 w321] -> w303
      tunnel: w301 -> [w319 w321]
      frame True {
        n109 = VISA Read(VISA resource name=w320, byte count=u32 1000, error in (no error)=w319) -> (VISA resource name out=w318:refnum<visa-resource-name>, read buffer=w315:string, error out=w317:errorcluster)  [unwired: 1 out]
        n110 = Decimal String To Number(string=w315) -> (number=w311:i32)  [unwired: 2 in, 1 out]
        "Sensor Raw Value 2" <- w311
        n111 = call <vilib>:"Median PtByPt.vi"("sample length"=20, "x"=w311) -> ("median"=w312:dbl)  [unwired: 2 in, 1 out]
        n112 = To Double Precision Float(number=w312) -> (double precision float=w308:dbl)
        n113 = Multiply(x=w308, y=0.0238) -> (x*y=w307:dbl)
        "Force in Kilograms" <- w307
        n114 = Multiply(x=w307, y=9.81) -> (x*y=→"Force in Newtons":dbl)
      }
      frame False {
      }
    }
    n115 = Or(x=w303, y=FALSE) -> (x .or. y?=w304:bool)
    n116 = Wait (ms)(milliseconds to wait=u32 5) -> ()  [unwired: 1 out]
  }
  n117 = VISA Close(VISA resource name=w71, error in (no error)=w72) -> (error out=w73:errorcluster)
  n118 = call <vilib>:"Simple Error Handler.vi"("error in (no error)"=w73) -> ()  [unwired: 1 in, 8 out]
  n119 = VISA Close(VISA resource name=w39, error in (no error)=w66) -> (error out=w67:errorcluster)
  n120 = call <vilib>:"Simple Error Handler.vi"("error in (no error)"=w67) -> ()  [unwired: 1 in, 8 out]
  n121 = stacked-sequence {
    tunnel: [_ w328] -> w46
    tunnel: [_ w327] -> w45
    frame #0 {
      w323 = 0
      w324 = FALSE
      w325 = ""
      # "Initialize Indicators"
      "Connected" <- w324
      "Start Time Text" <- w325
      "Stop Time Text" <- w325
      "Elapsed Time Text" <- w325
      "HostFrameCount" <- w323
      "Running" <- w324
      "Loop Iter" <- w323
      "PnoData" <- w324
    }
    frame #1 {
      # "Connect To Tracker"
      # "2. Initialize Tracker Connection"
      n122 = call <instrlib>:"PDI initialize.vi"() -> ("error out"=w327:errorcluster, "Connected"=w326:bool, "pDev"=w328:u32)  [unwired: 1 in, 4 out]
      n123 = local write "Connected"(w326) -> ()
    }
  }
  n124 = while {
    stop <- FALSE stop-if-true
    # "TRACKER 4"
    # "TRACKER 3"
    # "TRACKER 2"
    # "TRACKER 1"
    n125 = Index Array(array="XYZAER", index #1=0 ("index"), index #2=1 ("index"), index #3=2 ("index"), index #4=3 ("index")) -> (element #1=w336:T8, element #2=w362:T8, element #3=w361:T8, element #4=w360:T8)
    n126 = Unbundle By Name(w336) -> ("x"=w334:sgl, "y"=w332:sgl, "z"=w330:sgl)
    n127 = Unbundle By Name(w362) -> ("x"=w346:sgl, "y"=w345:sgl, "z"=w344:sgl)
    n128 = Multiply(x=w332, y=sgl -1.0) -> (x*y=w354:sgl)
    n129 = Multiply(x=w345, y=-1.0) -> (x*y=w353:dbl)
    n130 = Bundle(w353, "x"=w346) -> (w349:cluster{dbl, "x":sgl})  [unwired: 1 in]
    n131 = Bundle(w354, "x"=w334) -> (w350:cluster{sgl, "x":sgl})  [unwired: 1 in]
    n132 = Unbundle By Name(w361) -> ("x"=w343:sgl, "y"=w342:sgl, "z"=w341:sgl)
    n133 = Unbundle By Name(w360) -> ("x"=w333:sgl, "y"=w331:sgl, "z"=w329:sgl)
    n134 = Multiply(x=w342, y=-1.0) -> (x*y=w352:dbl)
    n135 = Multiply(x=w331, y=-1.0) -> (x*y=w351:dbl)
    n136 = Bundle(w352, "x"=w343) -> (w348:cluster{dbl, "x":sgl})  [unwired: 1 in]
    n137 = Bundle(w351, "x"=w333) -> (w347:cluster{dbl, "x":sgl})  [unwired: 1 in]
    n138 = Build Array(w350, w349, w348, w347) -> (→"Position Sensor Data":cluster{dbl, "x":sgl}[])
    n139 = Bundle("x"=w346, "y"=w345, "z"=w344) -> (→"Tracker 2 - X,Y,Z":cluster{"x":sgl, "y":sgl, "z":sgl})  [unwired: 1 in]
    n140 = Bundle("x"=w334, "y"=w332, "z"=w330) -> (→"Tracker 1 - X,Y,Z":cluster{"x":sgl, "y":sgl, "z":sgl})  [unwired: 1 in]
    n141 = Bundle("x"=w343, "y"=w342, "z"=w341) -> (→"Tracker 3 - X,Y,Z":cluster{"x":sgl, "y":sgl, "z":sgl})  [unwired: 1 in]
    n142 = Bundle("x"=w333, "y"=w331, "z"=w329) -> (→"Tracker 4 - X,Y,Z":cluster{"x":sgl, "y":sgl, "z":sgl})  [unwired: 1 in]
  }
  n143 = call <instrlib>:"PDI util stationcount.vi"("error in (no error)"=w45, "pDev"=w46) -> ("error out"=w44:errorcluster, "dup pDev"=w43:u32, "MaxCount"=w41:i32)  [unwired: 7 out]
  n144 = call <instrlib>:"PDI config setbuffer.vi"("error in (no error)"=w44, "Max sensors"=w41, "FrameCount"=w42, "pDev"=w43) -> ("error out"=w53:errorcluster, "dup pDev"=w54:u32)  [unwired: 6 out]
  n145 = flat-sequence {
    tunnel: w59 -> [_]
    tunnel: [w368] -> w55
    frame #0 {
      # "Get Start Time"
      n146 = Get Date/Time In Seconds() -> (seconds since 1Jan1904=w369:timestamp)
      n147 = Format Date/Time String(seconds (now)=w369) -> (date/time string=w370:string)  [unwired: 2 out]
      n148 = local write "Start Time Text"(w370) -> ()
      n149 = To Double Precision Float(number=w369) -> (double precision float=w368:dbl)
    }
  }
  n150 = call <instrlib>:"PDI action startcont.vi"("error in (no error)"=w53, "pDev"=w54) -> ("error out"=w60:errorcluster, "Running"=w52:bool, "dup pDev"=w59:u32)  [unwired: 7 out]
  n151 = control-ref of="HostFrameCount"() -> (w50:refnum<vi>)
  n152 = local write "Running"(w52) -> ()
  n153 = control-ref of="stop"() -> (w58:refnum<vi>)
  n154 = control-ref of="XYZAER"() -> (w49:refnum<vi>)
  n155 = Obtain Queue(element data type=0.0) -> (queue out=w6:refnum<queue>)  [unwired: 4 in, 2 out]
  n156 = while {
    shift-left: 0.0 ("Plant Output") -> [w437]
    shift-right: [w432] -> _
    tunnel: w25 -> [_]
    shift-right: [w418] -> _
    shift-left: 0.01 -> [w416]
    shift-right: [w390] -> _
    shift-left: TRUE -> [w415]
    shift-right: [w392] -> _
    shift-left: w22 -> [w414]
    shift-right: [w417] -> _
    shift-left: w22 -> [w413]
    tunnel: [w387] -> w21
    tunnel: [w373] -> w1
    tunnel: w6 -> [w371]
    stop <- "Stop 8" stop-if-true
    w378 = 1 items=["one channel for each line", "one channel for all lines"] ("line grouping")
    w387 = 0.05 ("Sampling Time dt (s)")
    w396 = 1 items=["one channel for each line", "one channel for all lines"] ("line grouping")
    w404 = 0.5 ("x")
    w431 = T7 {"static gain"=2.5, "lag (s)"=2.5, "deadtime (s)"=0.01, "load"=0.0, "deadband"=0.0, "sensor noise"=0.0, "initial PV"=30.0, "plant noise"=0.0}  # Process parameters
    w433 = FALSE  # Integrator ?
    # "C."
    # "Inlet 11"
    # "Exhaust 2"
    # "B."
    # "A."
    # "A.Output to PWM Logic \nB. Simulated Plant\nC. Draw Chart"
    # "Main PID Loop Control"
    n157 = Dequeue Element(queue=w371) -> (element=w372:dbl)  [unwired: 2 in, 3 out]
    n158 = Multiply(x=w387, y=1000.0) -> (x*y=w430:dbl)
    n159 = Not(x="Autotune 8") -> (.not. x?=w434:bool)
    n160 = feedback #4() -> (w439:bool)  [unwired: 1 in]
    n161 = feedback-in #4("Autotune 8") -> ()
    n162 = Wait Until Next ms Multiple(millisecond multiple=w430) -> ()  [unwired: 1 out]
    n163 = Exclusive Or(1:w439, 2:"Autotune 8") -> (0:w438:bool)
    n164 = feedback #5() -> (w436:dbl)  [unwired: 1 in]
    n165 = Multiply(x=w372, y=-1000.0) -> (x*y=w420:dbl)
    n166 = call <vilib>:"Median PtByPt.vi"("sample length"="Median sample length 17", "x"=w420) -> ("median"=w419:dbl)  [unwired: 2 in, 1 out]
    n167 = Square(x=w419) -> (x^2=w427:dbl)
    n168 = Multiply(x=w419, y=-7.5945) -> (x*y=w423:dbl)
    n169 = Multiply(x=w427, y=0.0612) -> (x*y=w424:dbl)
    n170 = Add(x=w423, y=w424) -> (x+y=w422:dbl)
    n171 = Add(x=143.72, y=w422) -> (x+y=w385:dbl)
    n172 = case shown="False" "Autotune 8" {
      tunnel: w387 -> [w454 _]
      tunnel: [w443 w459] -> w392
      tunnel: w437 -> [_ w458]
      tunnel: "PID Gains 8" -> [w453 _]
      tunnel: "Reinitialize 8" -> [w450 _]
      tunnel: w438 -> [w452 w457]
      tunnel: w436 -> [_ w461]
      tunnel: w385 -> [w446 _]
      tunnel: "Set Point 2" -> [w445 _]
      frame False {
        # "This code is to have 'bumpless' transfer from autotuning"
        n173 = Not(x=w452) -> (.not. x?=w449:bool)
        n174 = And(x="Automatic 8", y=w449) -> (x .and. y?=w451:bool)
        n175 = call-poly <vilib>:"PID Advanced.vi"("setpoint"=w445, "auto? (T)"=w451, "manual control"="MV: 8", "process variable"=w446, "alpha"=10.0, "PID gains"=w453, "dt (s)"=w454, "reinitialize? (F)"=w450) -> ("output"=w443:dbl)  [unwired: 6 in, 1 out]
      }
      frame True {
        w464 = 10000 ("sample length")
        # "Buffering data for parameters estimation"
        n176 = call <vilib>:"Data Queue PtByPt.vi"("initial queue element"=w458, "initialize"=w457, "sample length"=w464, "input data point"=w458) -> ("Current Queue"=→"Control Output 8":dbl[])  [unwired: 3 in, 4 out]
        n177 = Select(t=0.0, s=w457, f="Excitation 8") -> (s? t:f=w462:dbl)
        n178 = Add(x=w461, y=w462) -> (x+y=w459:dbl)
        n179 = call <vilib>:"Data Queue PtByPt.vi"("initial queue element"=w459, "initialize"=w457, "sample length"=w464, "input data point"=w459) -> ("Current Queue"=→"Measurement 8":dbl[])  [unwired: 3 in, 4 out]
      }
    }
    n180 = feedback-in #5(w392, w434) -> ()
    n181 = Greater?(x=w385, y="M-2") -> (0:w373:bool)
    n182 = Add(x=w416, y=w404) -> (x+y=w405:dbl)
    n183 = Subtract(x=w416, y=w404) -> (x-y=w403:dbl)
    n184 = Equal?(x=w414, y=w392) -> (x = y?=w411:bool)
    n185 = Greater?(x=w392, y=w414) -> (0:w410:bool)
    n186 = Select(t=w415, s=w411, f=w410) -> (s? t:f=w390:bool)
    "PWM Output 8" <- w390
    n187 = call "Plant System.vi"("Integrator ?"=w433, "Plant Input"=w392, "dt (s)"=w387, "process parameters"=w431) -> ("Plant Output"=w432:dbl)  [unwired: 11 in]
    n188 = Increment(x="Set Point 2") -> (x+1=w409:dbl)
    n189 = Decrement(x="Set Point 2") -> (x-1=w408:dbl)
    n190 = Select(t=w405, s=w390, f=w403) -> (s? t:f=w418:dbl)
    n191 = Select(t=w409, s=w390, f=w408) -> (s? t:f=w407:dbl)
    n192 = Not(x=w390) -> (.not. x?=w389:bool)
    n193 = call-poly <vilib>:"DAQmx Create Virtual Channel.vi"("lines"=tag "cDAQ1Mod1/port0/line6", "line grouping"=w396) -> ("task out"=w398:refnum<k21>, "error out"=w397:errorcluster)  [unwired: 12 in]
    n194 = call-poly <vilib>:"DAQmx Create Virtual Channel.vi"("lines"=tag "cDAQ1Mod2/port0/line6", "line grouping"=w378) -> ("task out"=w380:refnum<k21>, "error out"=w379:errorcluster)  [unwired: 12 in]
    n195 = Build Array(w385, "Set Point 2", w407) -> (w406:dbl[])
    n196 = Initialize Array("INLET 2 ON/OFF 2", 1 ("dimension size")) -> (w375:bool[])
    n197 = Initialize Array(w389, 1 ("dimension size")) -> (w393:bool[])
    n198 = local write "MV: 8"(w392) -> ()
    n199 = Add(x=w413, y=w416) -> (x+y=w417:dbl)
    n200 = Build Array(w406) -> (→"Real time Data 2":dbl[][])
    n201 = call-poly <vilib>:"DAQmx Write.vi"("task/channels in"=w398, "auto start"=TRUE, "data"=w393, "error in"=w397) -> ("task out"=w400:refnum<k21>, "error out"=w401:errorcluster)  [unwired: 9 in, 1 out]
    n202 = call-poly <vilib>:"DAQmx Write.vi"("task/channels in"=w380, "auto start"=TRUE, "data"=w375, "error in"=w379) -> ("task out"=w382:refnum<k21>, "error out"=w383:errorcluster)  [unwired: 9 in, 1 out]
    n203 = call <vilib>:"DAQmx Clear Task.vi"("task in"=w400, "error in"=w401) -> ("error out"=w395:errorcluster)  [unwired: 13 in]
    n204 = call <vilib>:"DAQmx Clear Task.vi"("task in"=w382, "error in"=w383) -> ("error out"=w377:errorcluster)  [unwired: 13 in]
    n205 = call <vilib>:"Simple Error Handler.vi"("error in (no error)"=w395) -> ()  [unwired: 4 in, 5 out]
    n206 = call <vilib>:"Simple Error Handler.vi"("error in (no error)"=w377) -> ()  [unwired: 4 in, 5 out]
  }
  n207 = Obtain Queue(element data type=0.0) -> (queue out=w5:refnum<queue>)  [unwired: 4 in, 2 out]
  n208 = while {
    shift-left: 0.0 ("Plant Output") -> [w531]
    shift-right: [w526] -> _
    tunnel: w31 -> [_]
    shift-right: [w512] -> _
    shift-left: 0.01 -> [w510]
    shift-right: [w484] -> _
    shift-left: TRUE -> [w509]
    shift-right: [w486] -> _
    shift-left: w28 -> [w508]
    shift-right: [w511] -> _
    shift-left: w28 -> [w507]
    tunnel: [w481] -> w27
    tunnel: [w467] -> w13
    tunnel: w5 -> [w465]
    stop <- "Stop 7" stop-if-true
    w472 = 1 items=["one channel for each line", "one channel for all lines"] ("line grouping")
    w481 = 0.05 ("Sampling Time dt (s)")
    w490 = 1 items=["one channel for each line", "one channel for all lines"] ("line grouping")
    w498 = 0.5 ("x")
    w525 = T7 {"static gain"=2.5, "lag (s)"=2.5, "deadtime (s)"=0.01, "load"=0.0, "deadband"=0.0, "sensor noise"=0.0, "initial PV"=30.0, "plant noise"=0.0}  # Process parameters
    w527 = FALSE  # Integrator ?
    # "C."
    # "Inlet 11"
    # "Exhaust 7"
    # "B."
    # "A."
    # "A.Output to PWM Logic \nB. Simulated Plant\nC. Draw Chart"
    # "Main PID Loop Control"
    n209 = Dequeue Element(queue=w465) -> (element=w466:dbl)  [unwired: 2 in, 3 out]
    n210 = Multiply(x=w481, y=1000.0) -> (x*y=w524:dbl)
    n211 = Not(x="Autotune 7") -> (.not. x?=w528:bool)
    n212 = feedback #6() -> (w533:bool)  [unwired: 1 in]
    n213 = feedback-in #6("Autotune 7") -> ()
    n214 = Wait Until Next ms Multiple(millisecond multiple=w524) -> ()  [unwired: 1 out]
    n215 = Exclusive Or(1:w533, 2:"Autotune 7") -> (0:w532:bool)
    n216 = feedback #7() -> (w530:dbl)  [unwired: 1 in]
    n217 = Multiply(x=w466, y=-1000.0) -> (x*y=w514:dbl)
    n218 = call <vilib>:"Median PtByPt.vi"("sample length"="Median sample length 16", "x"=w514) -> ("median"=w513:dbl)  [unwired: 2 in, 1 out]
    n219 = Square(x=w513) -> (x^2=w521:dbl)
    n220 = Multiply(x=w513, y=-0.6707) -> (x*y=w517:dbl)
    n221 = Multiply(x=w521, y=0.0015) -> (x*y=w518:dbl)
    n222 = Add(x=w517, y=w518) -> (x+y=w516:dbl)
    n223 = Add(x=-0.8771, y=w516) -> (x+y=w479:dbl)
    n224 = case shown="False" "Autotune 7" {
      tunnel: w481 -> [w548 _]
      tunnel: [w537 w553] -> w486
      tunnel: w531 -> [_ w552]
      tunnel: "PID Gains 7" -> [w547 _]
      tunnel: "Reinitialize 7" -> [w544 _]
      tunnel: w532 -> [w546 w551]
      tunnel: w530 -> [_ w555]
      tunnel: w479 -> [w540 _]
      tunnel: "Set Point 7" -> [w539 _]
      frame False {
        # "This code is to have 'bumpless' transfer from autotuning"
        n225 = Not(x=w546) -> (.not. x?=w543:bool)
        n226 = And(x="Automatic 7", y=w543) -> (x .and. y?=w545:bool)
        n227 = call-poly <vilib>:"PID Advanced.vi"("setpoint"=w539, "auto? (T)"=w545, "manual control"="MV: 7", "process variable"=w540, "alpha"=10.0, "PID gains"=w547, "dt (s)"=w548, "reinitialize? (F)"=w544) -> ("output"=w537:dbl)  [unwired: 6 in, 1 out]
      }
      frame True {
        w558 = 10000 ("sample length")
        # "Buffering data for parameters estimation"
        n228 = call <vilib>:"Data Queue PtByPt.vi"("initial queue element"=w552, "initialize"=w551, "sample length"=w558, "input data point"=w552) -> ("Current Queue"=→"Control Output 7":dbl[])  [unwired: 3 in, 4 out]
        n229 = Select(t=0.0, s=w551, f="Excitation 7") -> (s? t:f=w556:dbl)
        n230 = Add(x=w555, y=w556) -> (x+y=w553:dbl)
        n231 = call <vilib>:"Data Queue PtByPt.vi"("initial queue element"=w553, "initialize"=w551, "sample length"=w558, "input data point"=w553) -> ("Current Queue"=→"Measurement 7":dbl[])  [unwired: 3 in, 4 out]
      }
    }
    n232 = feedback-in #7(w486, w528) -> ()
    n233 = Greater?(x=w479, y="M-7") -> (0:w467:bool)
    n234 = Add(x=w510, y=w498) -> (x+y=w499:dbl)
    n235 = Subtract(x=w510, y=w498) -> (x-y=w497:dbl)
    n236 = Equal?(x=w508, y=w486) -> (x = y?=w505:bool)
    n237 = Greater?(x=w486, y=w508) -> (0:w504:bool)
    n238 = Select(t=w509, s=w505, f=w504) -> (s? t:f=w484:bool)
    "PWM Output 7" <- w484
    n239 = call "Plant System.vi"("Integrator ?"=w527, "Plant Input"=w486, "dt (s)"=w481, "process parameters"=w525) -> ("Plant Output"=w526:dbl)  [unwired: 11 in]
    n240 = Increment(x="Set Point 7") -> (x+1=w503:dbl)
    n241 = Decrement(x="Set Point 7") -> (x-1=w502:dbl)
    n242 = Select(t=w499, s=w484, f=w497) -> (s? t:f=w512:dbl)
    n243 = Select(t=w503, s=w484, f=w502) -> (s? t:f=w501:dbl)
    n244 = Not(x=w484) -> (.not. x?=w483:bool)
    n245 = call-poly <vilib>:"DAQmx Create Virtual Channel.vi"("lines"=tag "cDAQ1Mod8/port0/line4", "line grouping"=w490) -> ("task out"=w492:refnum<k21>, "error out"=w491:errorcluster)  [unwired: 12 in]
    n246 = call-poly <vilib>:"DAQmx Create Virtual Channel.vi"("lines"=tag "cDAQ1Mod7/port0/line3", "line grouping"=w472) -> ("task out"=w474:refnum<k21>, "error out"=w473:errorcluster)  [unwired: 12 in]
    n247 = Build Array(w479, "Set Point 7", w501) -> (w500:dbl[])
    n248 = Initialize Array("INLET 7 ON/OFF 2", 1 ("dimension size")) -> (w469:bool[])
    n249 = Initialize Array(w483, 1 ("dimension size")) -> (w487:bool[])
    n250 = local write "MV: 7"(w486) -> ()
    n251 = Add(x=w507, y=w510) -> (x+y=w511:dbl)
    n252 = Build Array(w500) -> (→"Real time Data 7":dbl[][])
    n253 = call-poly <vilib>:"DAQmx Write.vi"("task/channels in"=w492, "auto start"=TRUE, "data"=w487, "error in"=w491) -> ("task out"=w494:refnum<k21>, "error out"=w495:errorcluster)  [unwired: 9 in, 1 out]
    n254 = call-poly <vilib>:"DAQmx Write.vi"("task/channels in"=w474, "auto start"=TRUE, "data"=w469, "error in"=w473) -> ("task out"=w476:refnum<k21>, "error out"=w477:errorcluster)  [unwired: 9 in, 1 out]
    n255 = call <vilib>:"DAQmx Clear Task.vi"("task in"=w494, "error in"=w495) -> ("error out"=w489:errorcluster)  [unwired: 13 in]
    n256 = call <vilib>:"DAQmx Clear Task.vi"("task in"=w476, "error in"=w477) -> ("error out"=w471:errorcluster)  [unwired: 13 in]
    n257 = call <vilib>:"Simple Error Handler.vi"("error in (no error)"=w489) -> ()  [unwired: 4 in, 5 out]
    n258 = call <vilib>:"Simple Error Handler.vi"("error in (no error)"=w471) -> ()  [unwired: 4 in, 5 out]
  }
  n259 = Obtain Queue(element data type=0.0) -> (queue out=w9:refnum<queue>)  [unwired: 4 in, 2 out]
  n260 = while {
    shift-left: 0.0 ("Plant Output") -> [w656]
    shift-right: [w651] -> _
    tunnel: w79 -> [_]
    shift-right: [w637] -> _
    shift-left: 0.01 -> [w635]
    shift-right: [w610] -> _
    shift-left: TRUE -> [w634]
    shift-right: [w612] -> _
    shift-left: w76 -> [w633]
    shift-right: [w636] -> _
    shift-left: w76 -> [w632]
    tunnel: [w607] -> w75
    tunnel: [w604] -> w2
    tunnel: w11 -> [w582]
    tunnel: w9 -> [w581]
    tunnel: w6 -> [w578]
    tunnel: w5 -> [w577]
    stop <- "Stop" stop-if-true
    w562 = 1 items=["one channel for each line", "one channel for all lines"] ("line grouping")
    w570 = 1 items=["one channel for each line", "one channel for all lines"] ("line grouping")
    w597 = 1 items=["one channel for each line", "one channel for all lines"] ("line grouping")
    w607 = 0.05 ("Sampling Time dt (s)")
    w615 = 1 items=["one channel for each line", "one channel for all lines"] ("line grouping")
    w623 = 0.5 ("x")
    w650 = T7 {"static gain"=2.5, "lag (s)"=2.5, "deadtime (s)"=0.01, "load"=0.0, "deadband"=0.0, "sensor noise"=0.0, "initial PV"=30.0, "plant noise"=0.0}  # Process parameters
    w652 = FALSE  # Integrator ?
    # "Inlet 11"
    # "Exhaust 12"
    # "C."
    # "Inlet 11"
    # "Exhaust 11"
    # "B."
    # "A."
    # "A.Output to PWM Logic \nB. Simulated Plant\nC. Draw Chart"
    # "Main PID Loop Control"
    n261 = call-poly <vilib>:"DAQmx Read.vi"("task/channels in"=refnum<k21> "1_4_2_7_6_5") -> ("data"=w587:dbl[])  [unwired: 12 in, 2 out]
    n262 = Index Array(array=w587, index=0) -> (element=w583:dbl)
    n263 = Index Array(array=w587, index=1) -> ()  [unwired: 1 out]
    n264 = Index Array(array=w587, index=2) -> (element=w580:dbl)
    n265 = Index Array(array=w587, index=5) -> (element=w585:dbl)
    n266 = Index Array(array=w587, index=4) -> (element=w584:dbl)
    n267 = Index Array(array=w587, index=3) -> (element=w579:dbl)
    n268 = Enqueue Element(queue=w581, element=w583) -> ()  [unwired: 2 in, 3 out]
    n269 = Enqueue Element(queue=w578, element=w580) -> ()  [unwired: 2 in, 3 out]
    n270 = Multiply(x=w607, y=1000.0) -> (x*y=w649:dbl)
    n271 = Not(x="Autotune") -> (.not. x?=w653:bool)
    n272 = feedback #8() -> (w658:bool)  [unwired: 1 in]
    n273 = feedback-in #8("Autotune") -> ()
    n274 = Enqueue Element(queue=w577, element=w579) -> ()  [unwired: 2 in, 3 out]
    n275 = Wait Until Next ms Multiple(millisecond multiple=w649) -> ()  [unwired: 1 out]
    n276 = Exclusive Or(1:w658, 2:"Autotune") -> (0:w657:bool)
    n277 = feedback #9() -> (w655:dbl)  [unwired: 1 in]
    n278 = Enqueue Element(queue=w582, element=w584) -> ()  [unwired: 2 in, 3 out]
    n279 = Multiply(x=w585, y=-1000.0) -> (x*y=w639:dbl)
    n280 = call <vilib>:"Median PtByPt.vi"("sample length"="Median sample length", "x"=w639) -> ("median"=w638:dbl)  [unwired: 2 in, 1 out]
    n281 = Square(x=w638) -> (x^2=w646:dbl)
    n282 = Multiply(x=w638, y=-39.646) -> (x*y=w642:dbl)
    n283 = Multiply(x=w646, y=0.2324) -> (x*y=w643:dbl)
    n284 = Add(x=w642, y=w643) -> (x+y=w641:dbl)
    n285 = Add(x=1678.0, y=w641) -> (x+y=w605:dbl)
    n286 = case shown="False" "Autotune" {
      tunnel: w607 -> [w673 _]
      tunnel: [w662 w678] -> w612
      tunnel: w656 -> [_ w677]
      tunnel: "PID Gains" -> [w672 _]
      tunnel: "Reinitialize" -> [w669 _]
      tunnel: w657 -> [w671 w676]
      tunnel: w655 -> [_ w680]
      tunnel: w605 -> [w665 _]
      tunnel: "Set Point 11,12" -> [w664 _]
      frame False {
        # "This code is to have 'bumpless' transfer from autotuning"
        n287 = Not(x=w671) -> (.not. x?=w668:bool)
        n288 = And(x="Automatic", y=w668) -> (x .and. y?=w670:bool)
        n289 = call-poly <vilib>:"PID Advanced.vi"("setpoint"=w664, "auto? (T)"=w670, "manual control"="MV:", "process variable"=w665, "alpha"=10.0, "PID gains"=w672, "dt (s)"=w673, "reinitialize? (F)"=w669) -> ("output"=w662:dbl)  [unwired: 6 in, 1 out]
      }
      frame True {
        w683 = 10000 ("sample length")
        # "Buffering data for parameters estimation"
        n290 = call <vilib>:"Data Queue PtByPt.vi"("initial queue element"=w677, "initialize"=w676, "sample length"=w683, "input data point"=w677) -> ("Current Queue"=→"Control Output":dbl[])  [unwired: 3 in, 4 out]
        n291 = Select(t=0.0, s=w676, f="Excitation") -> (s? t:f=w681:dbl)
        n292 = Add(x=w680, y=w681) -> (x+y=w678:dbl)
        n293 = call <vilib>:"Data Queue PtByPt.vi"("initial queue element"=w678, "initialize"=w676, "sample length"=w683, "input data point"=w678) -> ("Current Queue"=→"Measurement":dbl[])  [unwired: 3 in, 4 out]
      }
    }
    n294 = feedback-in #9(w612, w653) -> ()
    n295 = Greater?(x=w605, y="M-11,12") -> (0:w604:bool)
    n296 = Add(x=w635, y=w623) -> (x+y=w624:dbl)
    n297 = Subtract(x=w635, y=w623) -> (x-y=w622:dbl)
    n298 = Equal?(x=w633, y=w612) -> (x = y?=w630:bool)
    n299 = Greater?(x=w612, y=w633) -> (0:w629:bool)
    n300 = Select(t=w634, s=w630, f=w629) -> (s? t:f=w610:bool)
    "PWM Output" <- w610
    n301 = call "Plant System.vi"("Integrator ?"=w652, "Plant Input"=w612, "dt (s)"=w607, "process parameters"=w650) -> ("Plant Output"=w651:dbl)  [unwired: 11 in]
    n302 = Increment(x="Set Point 11,12") -> (x+1=w628:dbl)
    n303 = Decrement(x="Set Point 11,12") -> (x-1=w627:dbl)
    n304 = Select(t=w624, s=w610, f=w622) -> (s? t:f=w637:dbl)
    n305 = Select(t=w628, s=w610, f=w627) -> (s? t:f=w626:dbl)
    n306 = Not(x=w610) -> (.not. x?=w609:bool)
    n307 = call-poly <vilib>:"DAQmx Create Virtual Channel.vi"("lines"=tag "cDAQ1Mod1/port0/line2", "line grouping"=w615) -> ("task out"=w617:refnum<k21>, "error out"=w616:errorcluster)  [unwired: 12 in]
    n308 = call-poly <vilib>:"DAQmx Create Virtual Channel.vi"("lines"=tag "cDAQ1Mod2/port0/line2", "line grouping"=w597) -> ("task out"=w599:refnum<k21>, "error out"=w598:errorcluster)  [unwired: 12 in]
    n309 = Build Array(w605, "Set Point 11,12", w626) -> (w625:dbl[])
    n310 = Initialize Array("INLET", 1 ("dimension size")) -> (w559:bool[])
    n311 = Initialize Array(w609, 1 ("dimension size")) -> (w560:bool[])
    n312 = call-poly <vilib>:"DAQmx Create Virtual Channel.vi"("lines"=tag "cDAQ1Mod8/port0/line2", "line grouping"=w570) -> ("task out"=w572:refnum<k21>, "error out"=w571:errorcluster)  [unwired: 12 in]
    n313 = call-poly <vilib>:"DAQmx Create Virtual Channel.vi"("lines"=tag "cDAQ1Mod7/port0/line1", "line grouping"=w562) -> ("task out"=w564:refnum<k21>, "error out"=w563:errorcluster)  [unwired: 12 in]
    n314 = local write "MV:"(w612) -> ()
    n315 = Add(x=w632, y=w635) -> (x+y=w636:dbl)
    n316 = Build Array(w625) -> (→"Real time Data -11,12":dbl[][])
    n317 = call-poly <vilib>:"DAQmx Write.vi"("task/channels in"=w617, "auto start"=TRUE, "data"=w560, "error in"=w616) -> ("task out"=w619:refnum<k21>, "error out"=w620:errorcluster)  [unwired: 9 in, 1 out]
    n318 = call-poly <vilib>:"DAQmx Write.vi"("task/channels in"=w599, "auto start"=TRUE, "data"=w559, "error in"=w598) -> ("task out"=w601:refnum<k21>, "error out"=w602:errorcluster)  [unwired: 9 in, 1 out]
    n319 = call-poly <vilib>:"DAQmx Write.vi"("task/channels in"=w572, "auto start"=TRUE, "data"=w560, "error in"=w571) -> ("task out"=w574:refnum<k21>, "error out"=w575:errorcluster)  [unwired: 9 in, 1 out]
    n320 = call-poly <vilib>:"DAQmx Write.vi"("task/channels in"=w564, "auto start"=TRUE, "data"=w559, "error in"=w563) -> ("task out"=w566:refnum<k21>, "error out"=w567:errorcluster)  [unwired: 9 in, 1 out]
    n321 = call <vilib>:"DAQmx Clear Task.vi"("task in"=w619, "error in"=w620) -> ("error out"=w614:errorcluster)  [unwired: 13 in]
    n322 = call <vilib>:"DAQmx Clear Task.vi"("task in"=w601, "error in"=w602) -> ("error out"=w596:errorcluster)  [unwired: 13 in]
    n323 = call <vilib>:"DAQmx Clear Task.vi"("task in"=w574, "error in"=w575) -> ("error out"=w569:errorcluster)  [unwired: 13 in]
    n324 = call <vilib>:"DAQmx Clear Task.vi"("task in"=w566, "error in"=w567) -> ("error out"=w561:errorcluster)  [unwired: 13 in]
    n325 = call <vilib>:"Simple Error Handler.vi"("error in (no error)"=w614) -> ()  [unwired: 4 in, 5 out]
    n326 = call <vilib>:"Simple Error Handler.vi"("error in (no error)"=w596) -> ()  [unwired: 4 in, 5 out]
    n327 = call <vilib>:"Simple Error Handler.vi"("error in (no error)"=w569) -> ()  [unwired: 4 in, 5 out]
    n328 = call <vilib>:"Simple Error Handler.vi"("error in (no error)"=w561) -> ()  [unwired: 4 in, 5 out]
  }
  n329 = while {
    tunnel: w79 -> [_]
    tunnel: w75 -> [w687]
    stop <- w697 stop-if-true
    # "If dT and deadtime have similar values, the identification could evaluate deadtime as zero and this generates proportional gain equal to Inf. This code avoid gain changes in this situations."
    # "Autotuning Loop"
    n330 = local read "Control Output"() -> (w699:dbl[])
    n331 = local read "Measurement"() -> (w698:dbl[])
    n332 = case shown="\"Chien-Hrones-Reswick\"" "Control" {
      tunnel: w699 -> [w708 w716 w725 w734]
      tunnel: w698 -> [w707 w715 w724 w733]
      tunnel: [w706 w714 w723 w732] -> w686
      tunnel: [w705 w713 w722 w731] -> w685
      tunnel: w687 -> [w704 w712 w721 w730]
      tunnel: [w703 w711 w720 w729] -> w684
      tunnel: [w702 w710 w719 w728] -> w689
      tunnel: "Type of controller" -> [w701 w709 w718 w727]
      frame "Ziegler-Nichols", Default {
        n333 = call-poly <vilib>:"PID Autotuning Design.vi"("Ziegler-Nichols Speed"="Ziegler-Nichols speed", "Type of Controller"=w701, "dt (s)"=w704, "Response signal"=w707, "Stimulus signal"=w708) -> ("PID gains"=w702:T3, "response operating point"=w705:dbl, "stimulus operating point"=w706:dbl, "Plant Parameters"=w703:T5)  [unwired: 3 in]
      }
      frame "Cohen-Coon" {
        n334 = call-poly <vilib>:"PID Autotuning Design.vi"("Type of Controller"=w709, "dt (s)"=w712, "Response signal"=w715, "Stimulus signal"=w716) -> ("PID gains"=w710:T3, "response offset"=w713:dbl, "stimulus offset"=w714:dbl, "Plant Parameters"=w711:T5)  [unwired: 4 in]
      }
      frame "Chien-Hrones-Reswick" {
        n335 = call-poly <vilib>:"PID Autotuning Design.vi"("Tuning specifications"="Tuning specifications", "Type of Controller"=w718, "dt (s)"=w721, "Response signal"=w724, "Stimulus signal"=w725) -> ("PID gains"=w719:T3, "response offset"=w722:dbl, "stimulus offset"=w723:dbl, "Plant Parameters"=w720:T5)  [unwired: 3 in]
      }
      frame "Internal Model Control" {
        n336 = call-poly <vilib>:"PID Autotuning Design.vi"("Desired Time Constant (tau_c)"="Multiplicative factor", "Type of Controller"=w727, "dt (s)"=w730, "Response signal"=w733, "Stimulus signal"=w734) -> ("PID gains"=w728:T3, "response offset"=w731:dbl, "stimulus offset"=w732:dbl, "Plant Parameters"=w729:T5)  [unwired: 3 in]
      }
    }
    "Stimulus operating point" <- w686
    "Response operating point" <- w685
    "Identified Plant Parameters" <- w684
    n337 = Unbundle(w689) -> ("proportional gain (Kc)"=w692:dbl)  [unwired: 2 out]
    n338 = Equal?(x=w692, y=inf) -> (x = y?=w691:bool)
    n339 = feedback #10() -> (w690:T3)  [unwired: 1 in]
    n340 = Select(t=w690, s=w691, f=w689) -> (s? t:f=w688:T3)
    "Tuned PID gains" <- w688
    n341 = feedback-in #10(w688) -> ()
    n342 = case shown="True" "Accept gain" {
      tunnel: w688 -> [_ w735]
      frame False {
      }
      frame True {
        n343 = local write "PID Gains"(w735) -> ()
      }
    }
    n344 = local read "Stop"() -> (w697:bool)
  }
  n345 = while {
    shift-left: 0.0 ("Plant Output") -> [w852]
    shift-right: [w847] -> _
    tunnel: w19 -> [_]
    shift-right: [w833] -> _
    shift-left: 0.01 -> [w831]
    shift-right: [w806] -> _
    shift-left: TRUE -> [w830]
    shift-right: [w808] -> _
    shift-left: w16 -> [w829]
    shift-right: [w832] -> _
    shift-left: w16 -> [w828]
    tunnel: [w803] -> w15
    tunnel: [w791] -> w4
    tunnel: w9 -> [w789]
    stop <- "Stop 12" stop-if-true
    w739 = 1 items=["one channel for each line", "one channel for all lines"] ("line grouping")
    w747 = 1 items=["one channel for each line", "one channel for all lines"] ("line grouping")
    w755 = 1 items=["one channel for each line", "one channel for all lines"] ("line grouping")
    w763 = 1 items=["one channel for each line", "one channel for all lines"] ("line grouping")
    w774 = 1 items=["one channel for each line", "one channel for all lines"] ("line grouping")
    w782 = 1 items=["one channel for each line", "one channel for all lines"] ("line grouping")
    w794 = 1 items=["one channel for each line", "one channel for all lines"] ("line grouping")
    w803 = 0.05 ("Sampling Time dt (s)")
    w811 = 1 items=["one channel for each line", "one channel for all lines"] ("line grouping")
    w819 = 0.5 ("x")
    w846 = T7 {"static gain"=2.5, "lag (s)"=2.5, "deadtime (s)"=0.01, "load"=0.0, "deadband"=0.0, "sensor noise"=0.0, "initial PV"=30.0, "plant noise"=0.0}  # Process parameters
    w848 = FALSE  # Integrator ?
    # "Inlet 11"
    # "Exhaust 3"
    # "Inlet 11"
    # "Exhaust 4"
    # "Inlet 11"
    # "Exhaust 5"
    # "C."
    # "Inlet 11"
    # "Exhaust 1"
    # "B."
    # "A."
    # "A.Output to PWM Logic \nB. Simulated Plant\nC. Draw Chart"
    # "Main PID Loop Control"
    n346 = Dequeue Element(queue=w789) -> (element=w790:dbl)  [unwired: 2 in, 3 out]
    n347 = Multiply(x=w803, y=1000.0) -> (x*y=w845:dbl)
    n348 = Not(x="Autotune 12") -> (.not. x?=w849:bool)
    n349 = feedback #11() -> (w854:bool)  [unwired: 1 in]
    n350 = feedback-in #11("Autotune 12") -> ()
    n351 = Wait Until Next ms Multiple(millisecond multiple=w845) -> ()  [unwired: 1 out]
    n352 = Exclusive Or(1:w854, 2:"Autotune 12") -> (0:w853:bool)
    n353 = feedback #12() -> (w851:dbl)  [unwired: 1 in]
    n354 = Multiply(x=w790, y=-1000.0) -> (x*y=w835:dbl)
    n355 = call <vilib>:"Median PtByPt.vi"("sample length"="Median sample length 21", "x"=w835) -> ("median"=w834:dbl)  [unwired: 2 in, 1 out]
    n356 = Square(x=w834) -> (x^2=w842:dbl)
    n357 = Multiply(x=w834, y=2.7367) -> (x*y=w838:dbl)
    n358 = Multiply(x=w842, y=0.0108) -> (x*y=w839:dbl)
    n359 = Add(x=w838, y=w839) -> (x+y=w837:dbl)
    n360 = Add(x=-331.61, y=w837) -> (x+y=w801:dbl)
    n361 = case shown="True" "Autotune 12" {
      tunnel: w803 -> [w869 _]
      tunnel: [w858 w874] -> w808
      tunnel: w852 -> [_ w873]
      tunnel: "PID Gains 12" -> [w868 _]
      tunnel: "Reinitialize 12" -> [w865 _]
      tunnel: w853 -> [w867 w872]
      tunnel: w851 -> [_ w876]
      tunnel: w801 -> [w861 _]
      tunnel: "Set Point 1,5" -> [w860 _]
      frame False {
        # "This code is to have 'bumpless' transfer from autotuning"
        n362 = Not(x=w867) -> (.not. x?=w864:bool)
        n363 = And(x="Automatic 12", y=w864) -> (x .and. y?=w866:bool)
        n364 = call-poly <vilib>:"PID Advanced.vi"("setpoint"=w860, "auto? (T)"=w866, "manual control"="MV: 12", "process variable"=w861, "alpha"=10.0, "PID gains"=w868, "dt (s)"=w869, "reinitialize? (F)"=w865) -> ("output"=w858:dbl)  [unwired: 6 in, 1 out]
      }
      frame True {
        w879 = 10000 ("sample length")
        # "Buffering data for parameters estimation"
        n365 = call <vilib>:"Data Queue PtByPt.vi"("initial queue element"=w873, "initialize"=w872, "sample length"=w879, "input data point"=w873) -> ("Current Queue"=→"Control Output 12":dbl[])  [unwired: 3 in, 4 out]
        n366 = Select(t=0.0, s=w872, f="Excitation 12") -> (s? t:f=w877:dbl)
        n367 = Add(x=w876, y=w877) -> (x+y=w874:dbl)
        n368 = call <vilib>:"Data Queue PtByPt.vi"("initial queue element"=w874, "initialize"=w872, "sample length"=w879, "input data point"=w874) -> ("Current Queue"=→"Measurement 12":dbl[])  [unwired: 3 in, 4 out]
      }
    }
    n369 = feedback-in #12(w808, w849) -> ()
    n370 = Greater?(x=w801, y="M-1,5") -> (0:w791:bool)
    n371 = Add(x=w831, y=w819) -> (x+y=w820:dbl)
    n372 = Subtract(x=w831, y=w819) -> (x-y=w818:dbl)
    n373 = Equal?(x=w829, y=w808) -> (x = y?=w826:bool)
    n374 = Greater?(x=w808, y=w829) -> (0:w825:bool)
    n375 = Select(t=w830, s=w826, f=w825) -> (s? t:f=w806:bool)
    "PWM Output 12" <- w806
    n376 = call "Plant System.vi"("Integrator ?"=w848, "Plant Input"=w808, "dt (s)"=w803, "process parameters"=w846) -> ("Plant Output"=w847:dbl)  [unwired: 11 in]
    n377 = Increment(x="Set Point 1,5") -> (x+1=w824:dbl)
    n378 = Decrement(x="Set Point 1,5") -> (x-1=w823:dbl)
    n379 = Select(t=w820, s=w806, f=w818) -> (s? t:f=w833:dbl)
    n380 = Select(t=w824, s=w806, f=w823) -> (s? t:f=w822:dbl)
    n381 = Not(x=w806) -> (.not. x?=w805:bool)
    n382 = call-poly <vilib>:"DAQmx Create Virtual Channel.vi"("lines"=tag "cDAQ1Mod8/port0/line5", "line grouping"=w763) -> ("task out"=w765:refnum<k21>, "error out"=w764:errorcluster)  [unwired: 12 in]
    n383 = call-poly <vilib>:"DAQmx Create Virtual Channel.vi"("lines"=tag "cDAQ1Mod7/port0/line4", "line grouping"=w755) -> ("task out"=w757:refnum<k21>, "error out"=w756:errorcluster)  [unwired: 12 in]
    n384 = call-poly <vilib>:"DAQmx Create Virtual Channel.vi"("lines"=tag "cDAQ1Mod1/port0/line7", "line grouping"=w811) -> ("task out"=w813:refnum<k21>, "error out"=w812:errorcluster)  [unwired: 12 in]
    n385 = call-poly <vilib>:"DAQmx Create Virtual Channel.vi"("lines"=tag "cDAQ1Mod2/port0/line7", "line grouping"=w794) -> ("task out"=w796:refnum<k21>, "error out"=w795:errorcluster)  [unwired: 12 in]
    n386 = Build Array(w801, "Set Point 1,5", w822) -> (w821:dbl[])
    n387 = Initialize Array("INLET 1,5 ON/OFF 3", 1 ("dimension size")) -> (w736:bool[])
    n388 = Initialize Array(w805, 1 ("dimension size")) -> (w737:bool[])
    n389 = local write "MV: 12"(w808) -> ()
    n390 = Add(x=w828, y=w831) -> (x+y=w832:dbl)
    n391 = Build Array(w821) -> (→"Real time Data 1,5,3,4":dbl[][])
    n392 = call-poly <vilib>:"DAQmx Write.vi"("task/channels in"=w765, "auto start"=TRUE, "data"=w737, "error in"=w764) -> ("task out"=w767:refnum<k21>, "error out"=w768:errorcluster)  [unwired: 9 in, 1 out]
    n393 = call-poly <vilib>:"DAQmx Write.vi"("task/channels in"=w757, "auto start"=TRUE, "data"=w736, "error in"=w756) -> ("task out"=w759:refnum<k21>, "error out"=w760:errorcluster)  [unwired: 9 in, 1 out]
    n394 = call-poly <vilib>:"DAQmx Write.vi"("task/channels in"=w813, "auto start"=TRUE, "data"=w737, "error in"=w812) -> ("task out"=w815:refnum<k21>, "error out"=w816:errorcluster)  [unwired: 9 in, 1 out]
    n395 = call-poly <vilib>:"DAQmx Write.vi"("task/channels in"=w796, "auto start"=TRUE, "data"=w736, "error in"=w795) -> ("task out"=w798:refnum<k21>, "error out"=w799:errorcluster)  [unwired: 9 in, 1 out]
    n396 = call <vilib>:"DAQmx Clear Task.vi"("task in"=w767, "error in"=w768) -> ("error out"=w762:errorcluster)  [unwired: 13 in]
    n397 = call <vilib>:"DAQmx Clear Task.vi"("task in"=w759, "error in"=w760) -> ("error out"=w754:errorcluster)  [unwired: 13 in]
    n398 = call <vilib>:"DAQmx Clear Task.vi"("task in"=w815, "error in"=w816) -> ("error out"=w810:errorcluster)  [unwired: 13 in]
    n399 = call <vilib>:"DAQmx Clear Task.vi"("task in"=w798, "error in"=w799) -> ("error out"=w793:errorcluster)  [unwired: 13 in]
    n400 = call <vilib>:"Simple Error Handler.vi"("error in (no error)"=w762) -> ()  [unwired: 4 in, 5 out]
    n401 = call <vilib>:"Simple Error Handler.vi"("error in (no error)"=w754) -> ()  [unwired: 4 in, 5 out]
    n402 = call <vilib>:"Simple Error Handler.vi"("error in (no error)"=w810) -> ()  [unwired: 4 in, 5 out]
    n403 = call <vilib>:"Simple Error Handler.vi"("error in (no error)"=w793) -> ()  [unwired: 4 in, 5 out]
    n404 = call-poly <vilib>:"DAQmx Create Virtual Channel.vi"("lines"=tag "cDAQ1Mod8/port0/line7", "line grouping"=w747) -> ("task out"=w749:refnum<k21>, "error out"=w748:errorcluster)  [unwired: 12 in]
    n405 = call-poly <vilib>:"DAQmx Create Virtual Channel.vi"("lines"=tag "cDAQ1Mod7/port0/line6", "line grouping"=w739) -> ("task out"=w741:refnum<k21>, "error out"=w740:errorcluster)  [unwired: 12 in]
    n406 = call-poly <vilib>:"DAQmx Create Virtual Channel.vi"("lines"=tag "cDAQ1Mod1/port0/line5", "line grouping"=w782) -> ("task out"=w784:refnum<k21>, "error out"=w783:errorcluster)  [unwired: 12 in]
    n407 = call-poly <vilib>:"DAQmx Create Virtual Channel.vi"("lines"=tag "cDAQ1Mod2/port0/line5", "line grouping"=w774) -> ("task out"=w776:refnum<k21>, "error out"=w775:errorcluster)  [unwired: 12 in]
    n408 = Initialize Array("INLET 1,5 ON/OFF 3", 1 ("dimension size")) -> (w771:bool[])
    n409 = call-poly <vilib>:"DAQmx Write.vi"("task/channels in"=w749, "auto start"=TRUE, "data"=w737, "error in"=w748) -> ("task out"=w751:refnum<k21>, "error out"=w752:errorcluster)  [unwired: 9 in, 1 out]
    n410 = call-poly <vilib>:"DAQmx Write.vi"("task/channels in"=w741, "auto start"=TRUE, "data"=w736, "error in"=w740) -> ("task out"=w743:refnum<k21>, "error out"=w744:errorcluster)  [unwired: 9 in, 1 out]
    n411 = call-poly <vilib>:"DAQmx Write.vi"("task/channels in"=w784, "auto start"=TRUE, "data"=w737, "error in"=w783) -> ("task out"=w786:refnum<k21>, "error out"=w787:errorcluster)  [unwired: 9 in, 1 out]
    n412 = call-poly <vilib>:"DAQmx Write.vi"("task/channels in"=w776, "auto start"=TRUE, "data"=w771, "error in"=w775) -> ("task out"=w778:refnum<k21>, "error out"=w779:errorcluster)  [unwired: 9 in, 1 out]
    n413 = call <vilib>:"DAQmx Clear Task.vi"("task in"=w751, "error in"=w752) -> ("error out"=w746:errorcluster)  [unwired: 13 in]
    n414 = call <vilib>:"DAQmx Clear Task.vi"("task in"=w743, "error in"=w744) -> ("error out"=w738:errorcluster)  [unwired: 13 in]
    n415 = call <vilib>:"DAQmx Clear Task.vi"("task in"=w786, "error in"=w787) -> ("error out"=w781:errorcluster)  [unwired: 13 in]
    n416 = call <vilib>:"DAQmx Clear Task.vi"("task in"=w778, "error in"=w779) -> ("error out"=w773:errorcluster)  [unwired: 13 in]
    n417 = call <vilib>:"Simple Error Handler.vi"("error in (no error)"=w746) -> ()  [unwired: 4 in, 5 out]
    n418 = call <vilib>:"Simple Error Handler.vi"("error in (no error)"=w738) -> ()  [unwired: 4 in, 5 out]
    n419 = call <vilib>:"Simple Error Handler.vi"("error in (no error)"=w781) -> ()  [unwired: 4 in, 5 out]
    n420 = call <vilib>:"Simple Error Handler.vi"("error in (no error)"=w773) -> ()  [unwired: 4 in, 5 out]
  }
  n421 = Compound Arithmetic op=OR(w2, w3, w4, w1, w1, w13) -> (w14:bool)
  "?" <- w14
  n422 = case shown="True" w14 {
    frame False {
    }
    frame True {
      n423 = call <vilib>:"Beep.vi"("use system alert? (T)"=FALSE, "duration (msec)"=u32 2000, "frequency (Hz)"=u32 15000) -> ()  [unwired: 9 in]
    }
  }
  n424 = control-ref of="PnoData"() -> (w40:refnum<vi>)
  n425 = call <instrlib>:"PDI data xyzaer loop.vi"("Data Ready Refnum"=w40, "FrameCount Ctl Ref"=w50, "error in (no error)"=w60, "xyzaer array\nRefnum"=w49, "Stop Ctl Ref"=w58, "pDev"=w59) -> ("error out"=w47:errorcluster, "Loop Iter"=w51:i32, "dup pDev"=w48:u32)  [unwired: 3 out]
  n426 = local write "Loop Iter"(w51) -> ()
  n427 = local write "Stop 12"(w19) -> ()
  n428 = call <instrlib>:"PDI action stopcont.vi"("error in (no error)"=w47, "pDev"=w48) -> ("error out"=w56:errorcluster, "Running"=w61:bool, "dup pDev"=w62:u32)  [unwired: 7 out]
  n429 = local write "Stop 8"(w25) -> ()
  n430 = local write "Stop 7"(w31) -> ()
  n431 = local write "Running"(w61) -> ()
  n432 = case shown="No Error" w47 {
    tunnel: w55 -> [w883 _]
    frame No Error {
      # "Success up to here"
      n433 = call "Elapsed Time"("Set Start Time (s)"=w883) -> ("Present Text"=w885:string, "Elapsed Time Text"=w884:string)  [unwired: 4 in, 13 out]
      n434 = local write "Stop Time Text"(w885) -> ()
      n435 = local write "Elapsed Time Text"(w884) -> ()
    }
    frame Error {
      # "Error somewhere;\nStop Time is irrelevant"
    }
  }
  n436 = while {
    tunnel: w19 -> [_]
    tunnel: w15 -> [w889]
    stop <- w899 stop-if-true
    # "If dT and deadtime have similar values, the identification could evaluate deadtime as zero and this generates proportional gain equal to Inf. This code avoid gain changes in this situations."
    # "Autotuning Loop"
    n437 = local read "Control Output 12"() -> (w901:dbl[])
    n438 = local read "Measurement 12"() -> (w900:dbl[])
    n439 = case shown="\"Ziegler-Nichols\", Default" "Control 12" {
      tunnel: w901 -> [w910 w918 w927 w936]
      tunnel: w900 -> [w909 w917 w926 w935]
      tunnel: [w908 w916 w925 w934] -> w887
      tunnel: [w907 w915 w924 w933] -> w888
      tunnel: w889 -> [w906 w914 w923 w932]
      tunnel: [w905 w913 w922 w931] -> w886
      tunnel: [w904 w912 w921 w930] -> w891
      tunnel: "Type of controller 12" -> [w903 w911 w920 w929]
      frame "Ziegler-Nichols", Default {
        n440 = call-poly <vilib>:"PID Autotuning Design.vi"("Ziegler-Nichols Speed"="Ziegler-Nichols speed 12", "Type of Controller"=w903, "dt (s)"=w906, "Response signal"=w909, "Stimulus signal"=w910) -> ("PID gains"=w904:T3, "response operating point"=w907:dbl, "stimulus operating point"=w908:dbl, "Plant Parameters"=w905:T5)  [unwired: 3 in]
      }
      frame "Cohen-Coon" {
        n441 = call-poly <vilib>:"PID Autotuning Design.vi"("Type of Controller"=w911, "dt (s)"=w914, "Response signal"=w917, "Stimulus signal"=w918) -> ("PID gains"=w912:T3, "response offset"=w915:dbl, "stimulus offset"=w916:dbl, "Plant Parameters"=w913:T5)  [unwired: 4 in]
      }
      frame "Chien-Hrones-Reswick" {
        n442 = call-poly <vilib>:"PID Autotuning Design.vi"("Tuning specifications"="Tuning specifications 12", "Type of Controller"=w920, "dt (s)"=w923, "Response signal"=w926, "Stimulus signal"=w927) -> ("PID gains"=w921:T3, "response offset"=w924:dbl, "stimulus offset"=w925:dbl, "Plant Parameters"=w922:T5)  [unwired: 3 in]
      }
      frame "Internal Model Control" {
        n443 = call-poly <vilib>:"PID Autotuning Design.vi"("Desired Time Constant (tau_c)"="Multiplicative factor 12", "Type of Controller"=w929, "dt (s)"=w932, "Response signal"=w935, "Stimulus signal"=w936) -> ("PID gains"=w930:T3, "response offset"=w933:dbl, "stimulus offset"=w934:dbl, "Plant Parameters"=w931:T5)  [unwired: 3 in]
      }
    }
    "Identified Plant Parameters 12" <- w886
    "Response operating point 12" <- w888
    "Stimulus operating point 12" <- w887
    n444 = Unbundle(w891) -> ("proportional gain (Kc)"=w894:dbl)  [unwired: 2 out]
    n445 = Equal?(x=w894, y=inf) -> (x = y?=w893:bool)
    n446 = feedback #13() -> (w892:T3)  [unwired: 1 in]
    n447 = Select(t=w892, s=w893, f=w891) -> (s? t:f=w890:T3)
    "Tuned PID gains 12" <- w890
    n448 = feedback-in #13(w890) -> ()
    n449 = case shown="True" "Accept gain 12" {
      tunnel: w890 -> [_ w937]
      frame False {
      }
      frame True {
        n450 = local write "PID Gains 12"(w937) -> ()
      }
    }
    n451 = local read "Stop 12"() -> (w899:bool)
  }
  n452 = while {
    tunnel: w25 -> [_]
    tunnel: w21 -> [w941]
    stop <- w951 stop-if-true
    # "If dT and deadtime have similar values, the identification could evaluate deadtime as zero and this generates proportional gain equal to Inf. This code avoid gain changes in this situations."
    # "Autotuning Loop"
    n453 = local read "Control Output 8"() -> (w953:dbl[])
    n454 = local read "Measurement 8"() -> (w952:dbl[])
    n455 = case shown="\"Chien-Hrones-Reswick\"" "Control 8" {
      tunnel: w953 -> [w962 w970 w979 w988]
      tunnel: w952 -> [w961 w969 w978 w987]
      tunnel: [w960 w968 w977 w986] -> w940
      tunnel: [w959 w967 w976 w985] -> w939
      tunnel: w941 -> [w958 w966 w975 w984]
      tunnel: [w957 w965 w974 w983] -> w938
      tunnel: [w956 w964 w973 w982] -> w943
      tunnel: "Type of controller 8" -> [w955 w963 w972 w981]
      frame "Ziegler-Nichols", Default {
        n456 = call-poly <vilib>:"PID Autotuning Design.vi"("Ziegler-Nichols Speed"="Ziegler-Nichols speed 8", "Type of Controller"=w955, "dt (s)"=w958, "Response signal"=w961, "Stimulus signal"=w962) -> ("PID gains"=w956:T3, "response operating point"=w959:dbl, "stimulus operating point"=w960:dbl, "Plant Parameters"=w957:T5)  [unwired: 3 in]
      }
      frame "Cohen-Coon" {
        n457 = call-poly <vilib>:"PID Autotuning Design.vi"("Type of Controller"=w963, "dt (s)"=w966, "Response signal"=w969, "Stimulus signal"=w970) -> ("PID gains"=w964:T3, "response offset"=w967:dbl, "stimulus offset"=w968:dbl, "Plant Parameters"=w965:T5)  [unwired: 4 in]
      }
      frame "Chien-Hrones-Reswick" {
        n458 = call-poly <vilib>:"PID Autotuning Design.vi"("Tuning specifications"="Tuning specifications 8", "Type of Controller"=w972, "dt (s)"=w975, "Response signal"=w978, "Stimulus signal"=w979) -> ("PID gains"=w973:T3, "response offset"=w976:dbl, "stimulus offset"=w977:dbl, "Plant Parameters"=w974:T5)  [unwired: 3 in]
      }
      frame "Internal Model Control" {
        n459 = call-poly <vilib>:"PID Autotuning Design.vi"("Desired Time Constant (tau_c)"="Multiplicative factor 8", "Type of Controller"=w981, "dt (s)"=w984, "Response signal"=w987, "Stimulus signal"=w988) -> ("PID gains"=w982:T3, "response offset"=w985:dbl, "stimulus offset"=w986:dbl, "Plant Parameters"=w983:T5)  [unwired: 3 in]
      }
    }
    "Stimulus operating point 8" <- w940
    "Response operating point 8" <- w939
    "Identified Plant Parameters 8" <- w938
    n460 = Unbundle(w943) -> ("proportional gain (Kc)"=w946:dbl)  [unwired: 2 out]
    n461 = Equal?(x=w946, y=inf) -> (x = y?=w945:bool)
    n462 = feedback #14() -> (w944:T3)  [unwired: 1 in]
    n463 = Select(t=w944, s=w945, f=w943) -> (s? t:f=w942:T3)
    "Tuned PID gains 8" <- w942
    n464 = feedback-in #14(w942) -> ()
    n465 = case shown="True" "Accept gain 8" {
      tunnel: w942 -> [_ w989]
      frame False {
      }
      frame True {
        n466 = local write "PID Gains 8"(w989) -> ()
      }
    }
    n467 = local read "Stop 8"() -> (w951:bool)
  }
  n468 = while {
    tunnel: w31 -> [_]
    tunnel: w27 -> [w993]
    stop <- w1003 stop-if-true
    # "If dT and deadtime have similar values, the identification could evaluate deadtime as zero and this generates proportional gain equal to Inf. This code avoid gain changes in this situations."
    # "Autotuning Loop"
    n469 = local read "Control Output 7"() -> (w1005:dbl[])
    n470 = local read "Measurement 7"() -> (w1004:dbl[])
    n471 = case shown="\"Chien-Hrones-Reswick\"" "Control 7" {
      tunnel: w1005 -> [w1014 w1022 w1031 w1040]
      tunnel: w1004 -> [w1013 w1021 w1030 w1039]
      tunnel: [w1012 w1020 w1029 w1038] -> w992
      tunnel: [w1011 w1019 w1028 w1037] -> w991
      tunnel: w993 -> [w1010 w1018 w1027 w1036]
      tunnel: [w1009 w1017 w1026 w1035] -> w990
      tunnel: [w1008 w1016 w1025 w1034] -> w995
      tunnel: "Type of controller 7" -> [w1007 w1015 w1024 w1033]
      frame "Ziegler-Nichols", Default {
        n472 = call-poly <vilib>:"PID Autotuning Design.vi"("Ziegler-Nichols Speed"="Ziegler-Nichols speed 7", "Type of Controller"=w1007, "dt (s)"=w1010, "Response signal"=w1013, "Stimulus signal"=w1014) -> ("PID gains"=w1008:T3, "response operating point"=w1011:dbl, "stimulus operating point"=w1012:dbl, "Plant Parameters"=w1009:T5)  [unwired: 3 in]
      }
      frame "Cohen-Coon" {
        n473 = call-poly <vilib>:"PID Autotuning Design.vi"("Type of Controller"=w1015, "dt (s)"=w1018, "Response signal"=w1021, "Stimulus signal"=w1022) -> ("PID gains"=w1016:T3, "response offset"=w1019:dbl, "stimulus offset"=w1020:dbl, "Plant Parameters"=w1017:T5)  [unwired: 4 in]
      }
      frame "Chien-Hrones-Reswick" {
        n474 = call-poly <vilib>:"PID Autotuning Design.vi"("Tuning specifications"="Tuning specifications 7", "Type of Controller"=w1024, "dt (s)"=w1027, "Response signal"=w1030, "Stimulus signal"=w1031) -> ("PID gains"=w1025:T3, "response offset"=w1028:dbl, "stimulus offset"=w1029:dbl, "Plant Parameters"=w1026:T5)  [unwired: 3 in]
      }
      frame "Internal Model Control" {
        n475 = call-poly <vilib>:"PID Autotuning Design.vi"("Desired Time Constant (tau_c)"="Multiplicative factor 7", "Type of Controller"=w1033, "dt (s)"=w1036, "Response signal"=w1039, "Stimulus signal"=w1040) -> ("PID gains"=w1034:T3, "response offset"=w1037:dbl, "stimulus offset"=w1038:dbl, "Plant Parameters"=w1035:T5)  [unwired: 3 in]
      }
    }
    "Stimulus operating point 7" <- w992
    "Response operating point 7" <- w991
    "Identified Plant Parameters 7" <- w990
    n476 = Unbundle(w995) -> ("proportional gain (Kc)"=w998:dbl)  [unwired: 2 out]
    n477 = Equal?(x=w998, y=inf) -> (x = y?=w997:bool)
    n478 = feedback #15() -> (w996:T3)  [unwired: 1 in]
    n479 = Select(t=w996, s=w997, f=w995) -> (s? t:f=w994:T3)
    "Tuned PID gains 7" <- w994
    n480 = feedback-in #15(w994) -> ()
    n481 = case shown="True" "Accept gain 7" {
      tunnel: w994 -> [_ w1041]
      frame False {
      }
      frame True {
        n482 = local write "PID Gains 7"(w1041) -> ()
      }
    }
    n483 = local read "Stop 7"() -> (w1003:bool)
  }
  n484 = call <instrlib>:"PDI close.vi"("error in (no error)"=w56, "pDev"=w62) -> ("error out"=→"error out":errorcluster, "connected"=w57:bool)  [unwired: 8 out]
  n485 = local write "Connected"(w57) -> ()
